vi "XY_plot_gnuplot.vi"(1 "Job Directory":path=path "/G4_2_HD/Users/paulhayden/Documents/Projects/Westlakes_resolution") -> (2 "Saved Automatically?":bool, 3 "Tex Info String":string="set term epslatex\nset output \"Plot.eps\"\nset xlabel '$Distance~(m)$'\nset ylabel '$DF~(s/m^3)\\times10^6$'\nset samples 1000\nset pointsize 1.00\nset title '$B38~Centreline~Glc$' 0, 0\nset size 0.75,0.9\n\n#set key 450, -2.5833\n unset key\nset label 1 '~~~~~~~~~~~Angle~(deg)~=~0' at -100, -2.58\nset label 2 '~~~~~~~~~~~Height~(m)~=~5' at -100, -3.27\n set xrange [0 : 500] \n# set autoscale x \n set yrange [0.10000 : 7]\n# set autoscale y \n\nplot \"B38_Centreline_Glc.dat\" index 0 using 1:2 axes x1y1 title '$File=B38R~DDD.xls$' with points 1 1, \\\n\"B38_Centreline_Glc.dat\" index 1 using 1:2 axes x1y1 title '$File=B38R~DDD~1.xls$' with points 1 3", 4 "Plot data file":path)   [LabVIEW 2022 SP3]
uses:
  Gnuplot_Label.ctl
  gnuplotScriptComponents/gridlines.ctl
  gnuplotScriptComponents/legendAppearance.ctl
  gnuplotScriptComponents/alignment.ctl
  gnuplotScriptComponents/legendProperties.ctl
  gnuplotScriptComponents/at.ctl
  <vilib>/Analysis/baseanly.llb/Mean (DBL).vi
  <vilib>/Utility/error.llb/Trim Whitespace One-Sided.vi
  Results_plotter_Global.vi
  Data plotting/subVIs/Plot_Values_Global.vi
  <vilib>/Analysis/NI_AALBase.lvlib
  <vilib>/Analysis/NI_AALPro.lvlib
panel:
  in  "Show Re-Run Gnuplot?":bool
  in  "Tab Control":T1(tab)
  in  "Plot Title":u16(ring) items=["Title String Only", "Date:Sortable:", "Run:Command:File", "Run:Start Time:", "Run:Description:", "Row:Number:", "Row:Type:", "Row:Start:(sec)", "Row:Comment:", "Timestamp::", "Config::", "Config:Num:", "Errata::", "Omit::", "WD::", "WD.Pt::", "WD.Pt.Cfg::", "Point:ID:", "Point:Row:", "Legend0::", "Downrange:Distance:(ft)", "Point:Height:Num", "Point:Column:", "Legend1::", "-:MeasuredVariables:-----------", "--:VelocityStats:--", "U_{dem}:Nominal:(m/s)", "U_{ref}::(m/s)", "\\overline{U}::(m/s)", "U:corr:(m/s)", "\\overline{V}::(m/s)", "\\overline{W}::(m/s)", "\\overline{|UV|}::(m/s)", "\\overline{|UW|}::(m/s)", "\\overline{|UVW|}::(m/s)", "\\overline{\\theta}::(deg)", "\\sigma^2(U)::(m/s)^2", "\\sigma^2(V)::(m/s)^2", "\\sigma^2(W)::(m/s)^2", "\\sigma^2(|UV|)::(m/s)^2", "\\sigma^2(|UW|)::(m/s)^2", "\\sigma^2(|UVW|)::(m/s)^2", "\\sigma^2(\\theta)::(deg^2)", "u'v'::(m^2/s^2)", "v'w'::(m^2/s^2)", "u'w'::(m^2/s^2)", "--:VelocityStatsEnd:--", "--:QAstats:--", "Omni:meanPSU:(V)", "Omni:varPSU:(V^2)", "Temp::(C)", "No Of:Measurement:Blocks", "No of:Analogue:Samples", "Flow:Measurement:Time", "Decimation::", "AFRaw:nGood:perDecBlock", "AFGoodV:nGood:perDecBlock", "AFGoodVP:nGood:perDecBlock", "AFRaw:nCone<58:deg", "AFRaw:nCone<90:deg", "AFRaw:Cone<58:deg", "AFRaw:Cone<90:deg", "Run:Messages:", "--:QAstatsEnd:--", "-:MeasuredVariablesEnd:-----------", "Max:(ConeAngle):(deg)", "Valid:AFReduction:Fraction", "Valid:Velocity:Fraction", "Valid:5hpPressure:Fraction", "-:LocationsStart:-------------", "Scale::", "Row:X:0", "X::(mm)", "Y::(mm)", "Z:(mm):", "U_{ref}:Z:(mm)", "Metadata:Motor:X", "Metadata:Motor:Y", "Metadata:Motor:Z", "-:LocationsEnd:-------------", "-:BLsetupBlock:------------", "BLS:Trip[1]:Ach(mm)", "BLS:Trip[2]:Ach(mm)", "BLS:Spires[1]:Ach(mm)", "BLS:Spires[2]:Ach(mm)", "BLS:Main[1]:Ach(mm)", "BLS:Main[2]:Ach(mm)", "BLS:Main[3]:Ach(mm)", "BLS:Boost[1]:Ach(mm)", "BLS:Boost[2]:Ach(mm)", "BLS:Boost[3]:Ach(mm)", "Main:Avg:(mm)", "Boost:Avg:(mm)", "FORMATTED:OUTPUT:BELOW-THIS-------------", "Configuration::", "Wind:Direction:(deg)", "BL:Setup:", "PointID::", "GDE:Uref:(m/s)", "Uref::(m/s)", "Mean:U:/U_{ref}", "Mean:V:/U_{ref}", "Mean:W:/U_{ref}", "Mean:|UV|:/U_{ref}", "Mean:|UW|:/U_ref", "Mean:|UVW|:/U_ref", "Yaw:(UV):(deg)", "TI:(U):(/U)", "TI:(U):(/|UV|)", "TI:(V):(/|UV|)", "TI:(W):(/|UW|)", "TI:(|UV|):(/|UV|)", "TI:(|UW|):(/|UW|)", "TI:(|UVW|):(/|UVW|)", "Velocity:Validation:(percent)", "Raw:Data:Filename", "FORMATTED:OUTPUT:ABOVE-THIS---------------", "Current:File:", "Current:Filepath:", "Template:File:Used", "Seconds:since:1st Jan", "Ramp:Request:0", "Ramp:Request:1", "Ramp:Request:2", "Ramp:Request:3", "Ramp:Request:4", "Ramp:Request:5", "Ramp:Request:6", "Ramp:Request:7", "Ramp:Request:8", "Ramp:Request:9", "Ramp:Request:10", "Ramp:Request:11", "Ramp:Request:12", "Point:Row:Column", "Number:of:Measurements"]
  in  "Plot Title":string
  in  "Added labels":i32[](listbox)
  in  "Show Labels?":bool
  in  "Summarise":u16(ring) items=["All Series", "\\overline{U} (m/s)", "GDE Uref (m/s)"]
  in  "X Log?":bool
  in  "Y Log?":bool
  in  "Ymin Val":dbl
  in  "Ymin":bool=TRUE
  in  "Xmin Val":dbl
  in  "Xmin":bool=TRUE
  in  "Xmax Val":dbl
  in  "Xmax":bool=TRUE
  in  "Ymax Val":dbl
  in  "Ymax":bool=TRUE
  in  "Major Gridlines":T2
  in  "Minor Gridlines":T2
  out "Time format?":bool
  in  "precision":string
  out "Profile offset":dbl
  in  "Offset?":bool
  in  "Mode":T3
  in  "Separation":dbl=1.2
  in  "Fit Line Width":i32=2
  in  "Fit type":T4(ring)
  in  "Put Coeff\nin Results file":bool
  in  "Analysis":T5(ring)
  in  "Wavelength?":bool
  in  "Auto Zp":bool=TRUE
  in  "Fixed Zp":dbl format="%.2f"
  in  "Something about fit..!":bool
  in  "Fit Line Type":i32=2
  in  "Current Fit Formula":string
  in  "Black and white?":bool
  in  "plot error bars?":bool
  in  "Plot style":u16[](array[ring])=[0, 0, 0, 0, 0, 0, 0, 0, 0, 0, 0] items=["points", "lines", "linespoints"]
  in  "Point Size":dbl=1.2 format="%.2f"
  in  "Graph Height":string="0.9"
  in  "Graph width":string="0.75"
  in  "Reverse order":bool
  in  "Appearance":T6
  in  "Show legend?":bool
  in  "Legend Position":u16(ring) items=["LabVIEW calculated", "top left", "top right", "bottom left", "bottom right", "below", "inside"]
  in  "Alignment":T7={"Horizontal"="center", "Vertical"="bottom"}
  in  "Save data analysis file":bool
  out "Path":path
  in  "Filename Max length":i32=28
  out "With legend":i32=580
  out "No Legend":i32=397
  out "No of Series":i32=2
  out "X location":dbl=-100.0
  out "Y location":dbl=-2.583333333333333
  out "Delta y":dbl=0.6900000000000001
  out "Extra range":dbl
  out "Final Title":string="B38 Centreline Glc"
  out "XY Graph":cluster{dbl[], dbl[]}[](graph)=[{[215.0, 270.0, 320.0, 445.0, 500.0, 500.0, 525.0, 600.0, 675.0, 750.0, 825.0, 900.0, 953.54, 960.0, 1010.0, 1060.0], [0.1374656, 0.6662545, 1.465458, 3.619824, 4.614524, 4.54365, 4.848976, 5.887329, 5.940571, 6.152151, 5.717487, 5.600293, 5.818368, 5.40069, 5.154843, 5.121789]}, {[100.0, 150.0, 215.0, 270.0, 320.0, 445.0, 525.0, 600.0, 675.0, 750.0, 825.0, 900.0, 960.0, 1010.0, 1060.0], [0.002314715, -0.00693192, 0.120417, 0.6880509, 1.519176, 3.513709, 5.065183, 6.116033, 6.096773, 5.938465, 5.593788, 5.5597, 5.387002, 5.304077, 4.887903]}]
  # "Scales"
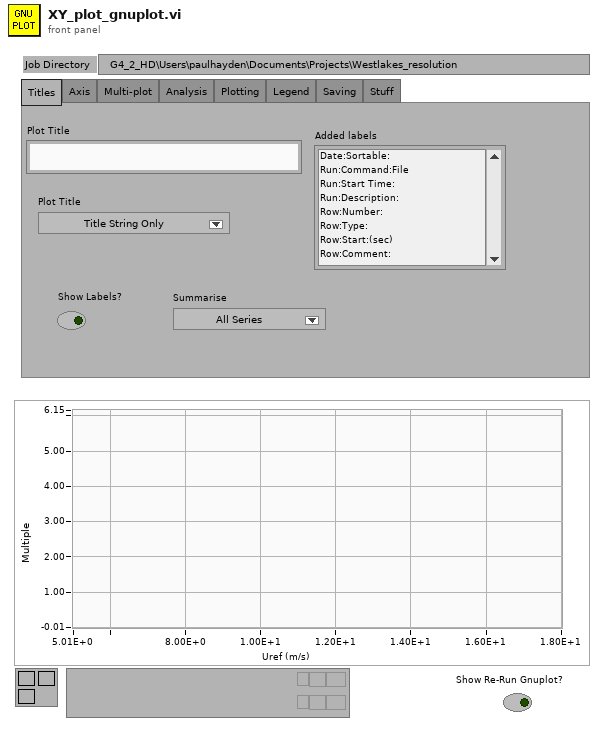
[diagram p1: front panel]
types:
  T1 = enum32{"Titles", "Axis", "Multi-plot", "Analysis", "Plotting", "Legend", "Saving", "Stuff"}
  T2 = typedef "gridlines.ctl" = enum16{"None", "X only", "Y only", "Both X and Y"}
  T3 = typedef "Gnuplot_Label.ctl" = enum16{"3 Labels per plot", "Only Center label", "Only Bottom Label"}
  T4 = enum16{"None", "Spline", "Linear", "2nd Poly", "3rd Poly", "4th Poly", "Gauss Lat", "Gauss vert", "Gauss Vert with 2 sig", "Guass glc"}
  T5 = enum16{"None", "% change", "Spectrum", "Norm Spec"}
  T6 = typedef "legendAppearance.ctl" = cluster{"layout":string, "text-sample order":string, "key order":string, "surroundingBox":string, "MaxRows":u32, "MaxCols":u32, "WidthAdjust":dbl}
  T7 = typedef "alignment.ctl" = cluster{"Horizontal":string, "Vertical":string}
  T8 = typedef "Error_bars.ctl" = cluster{"Upper":string[], "Lower":string[], "St Error":string[]}
  T9 = cluster{"Output":dbl[], "PercentageDifferenceArray":dbl[]}[]
  T10 = cluster{dbl[], "PercentageDifferenceArray":dbl[]}
  T11 = cluster{"Output":dbl[], "PercentageDifferenceArray":dbl[]}
  T12 = typedef "legendProperties.ctl" = cluster{"Appearance":T6, "Alignment":T7, "Location":string, "\"At\" location":T13}
  T13 = typedef "at.ctl" = cluster{"XcoordSys":string, "YcoordSys":string, "Xvalue":dbl, "Yvalue":dbl}
  T14 = typedef "RFP_Plot_Metadata.ctl" = cluster{"Row Number":i32[], "Error Bars":T15, "X Label":string, "Y Label":string, "Blanks NaNs":i32[]}
  T15 = typedef "Error_bars_index.ctl" = cluster{"Upper":i32, "Lower":i32, "St Error":i32}
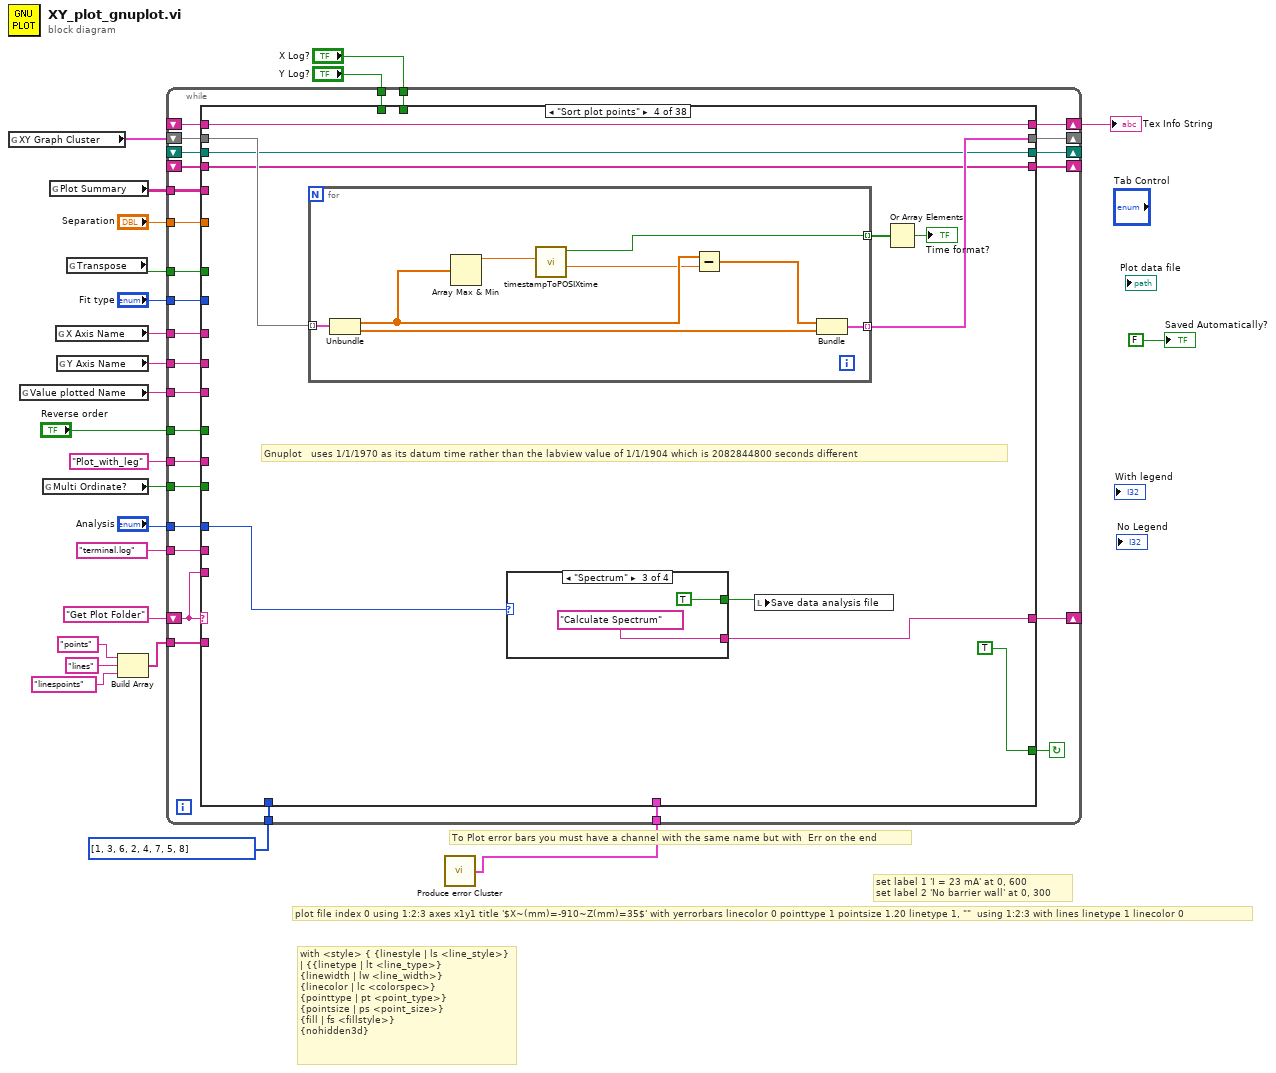
[diagram p0: block diagram]
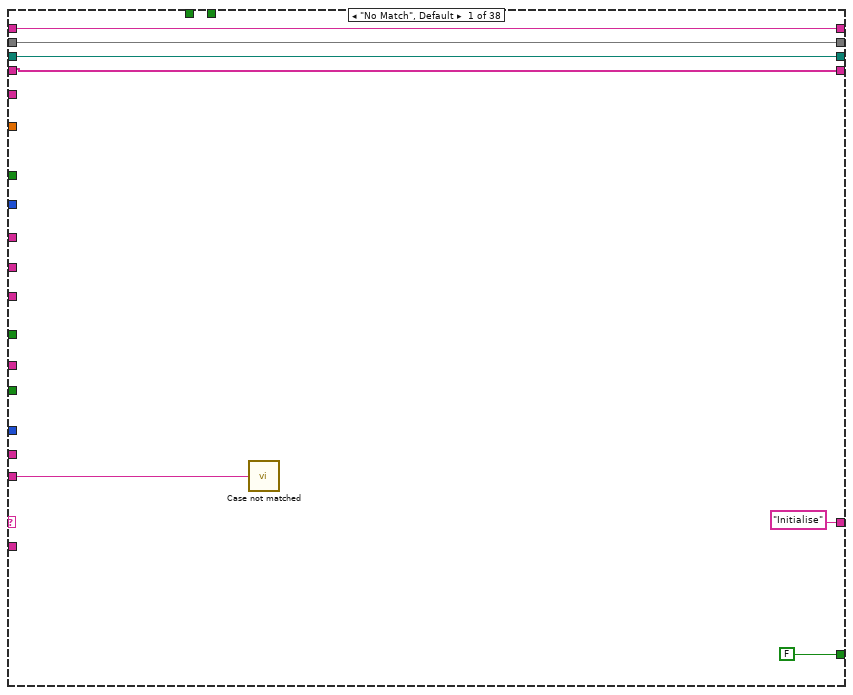
[diagram p2: hidden frame]
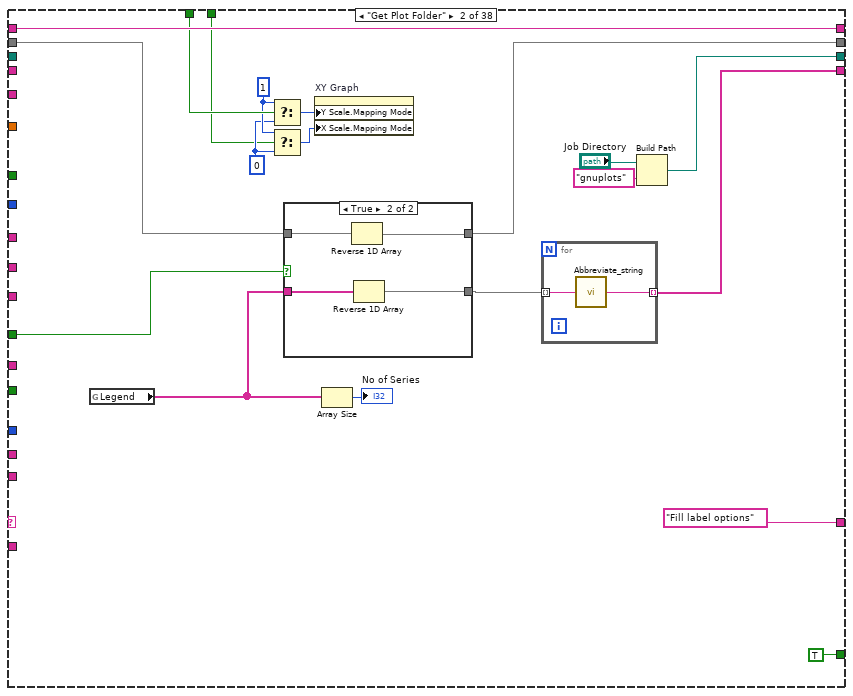
[diagram p3: hidden frame]
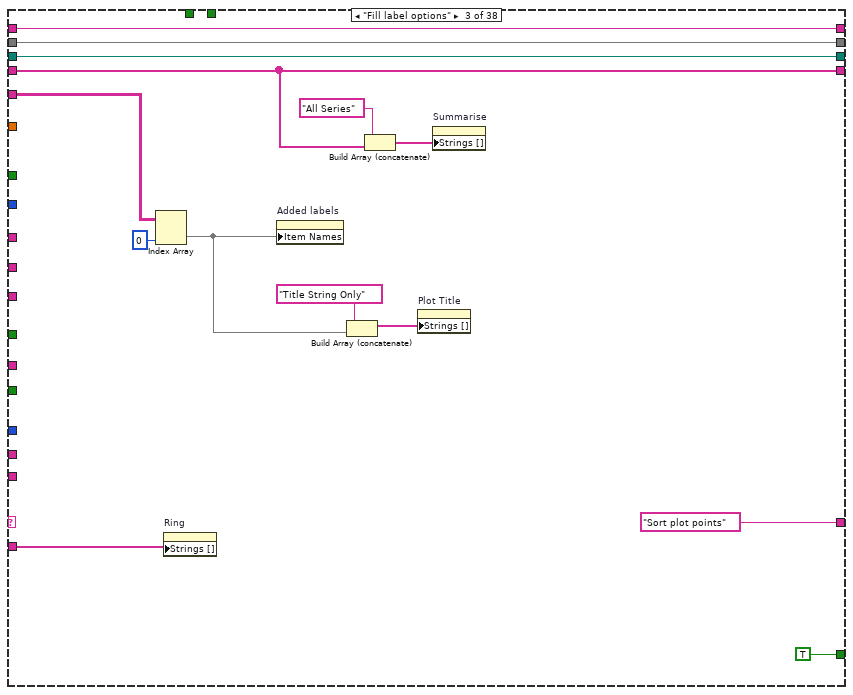
[diagram p5: hidden frame]
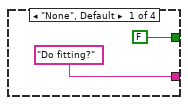
[diagram p6: hidden frame]
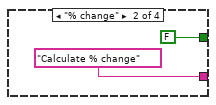
[diagram p7: hidden frame]
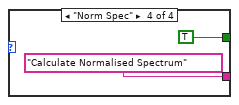
[diagram p8: hidden frame]
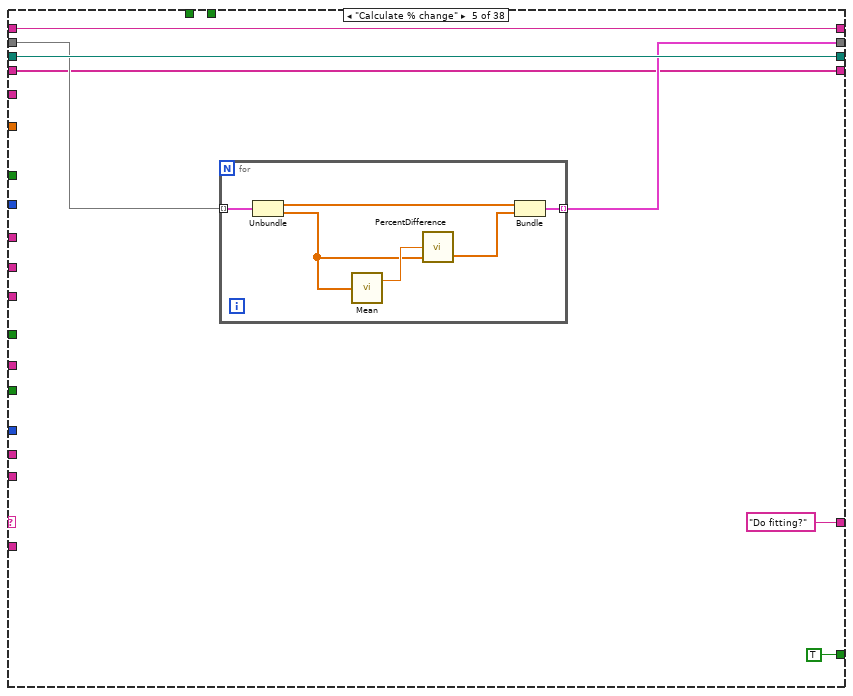
[diagram p9: hidden frame]
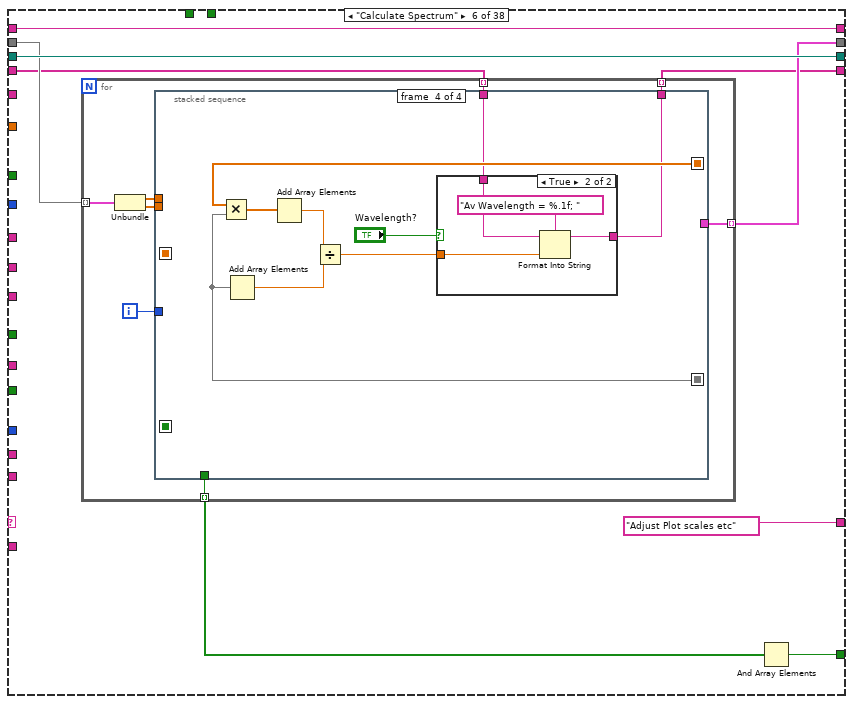
[diagram p10: hidden frame]
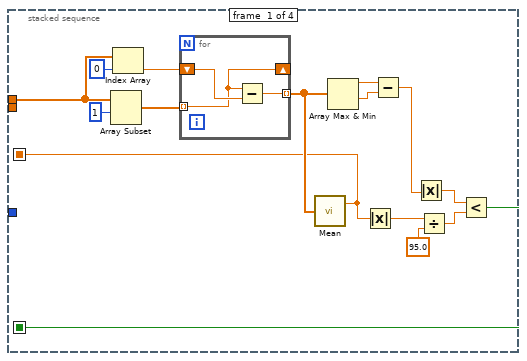
[diagram p11: hidden frame]
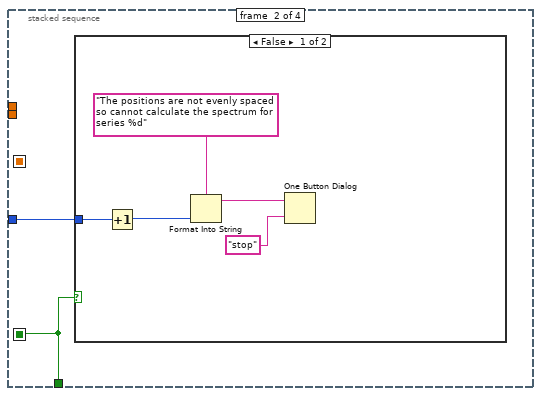
[diagram p12: hidden frame]
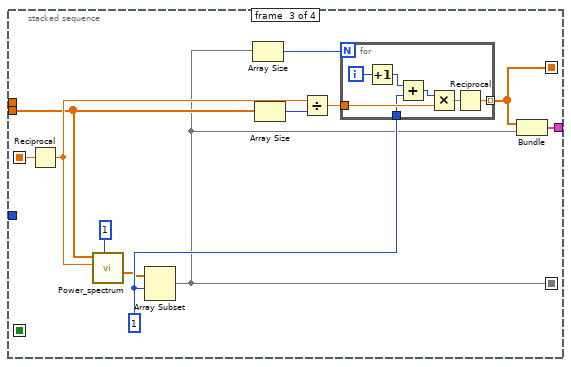
[diagram p14: hidden frame]
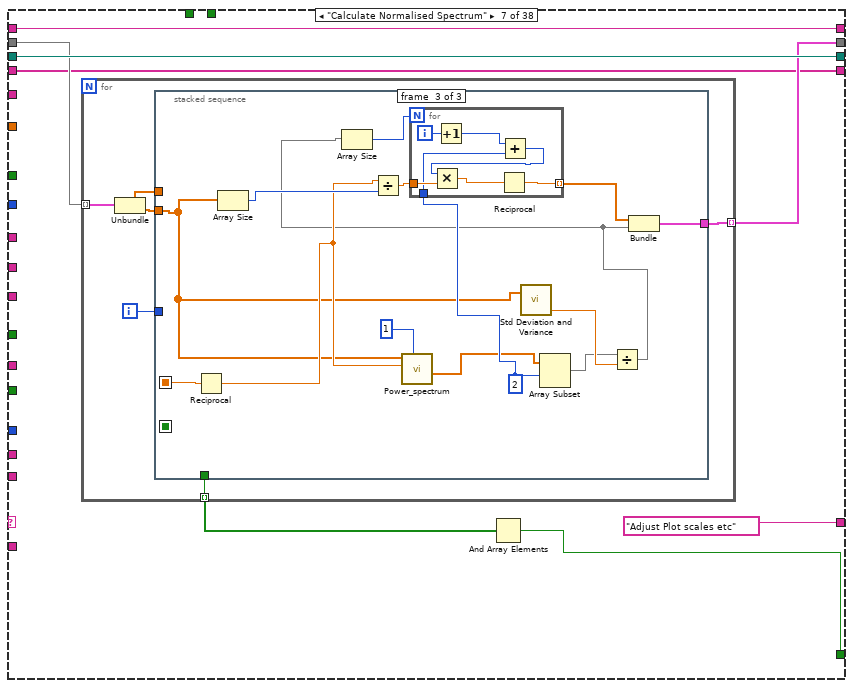
[diagram p16: hidden frame]
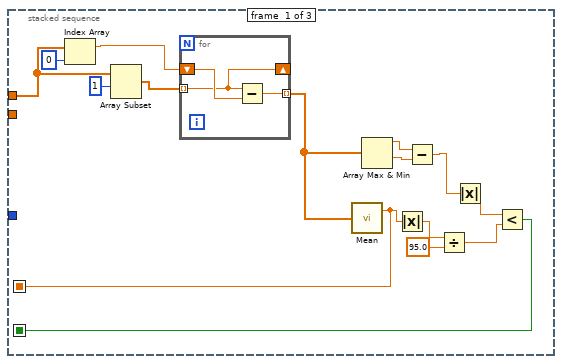
[diagram p17: hidden frame]
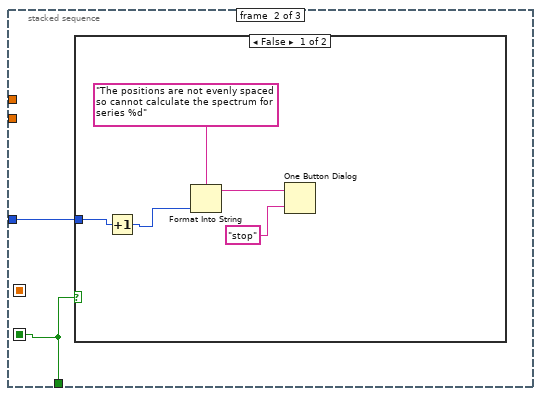
[diagram p18: hidden frame]
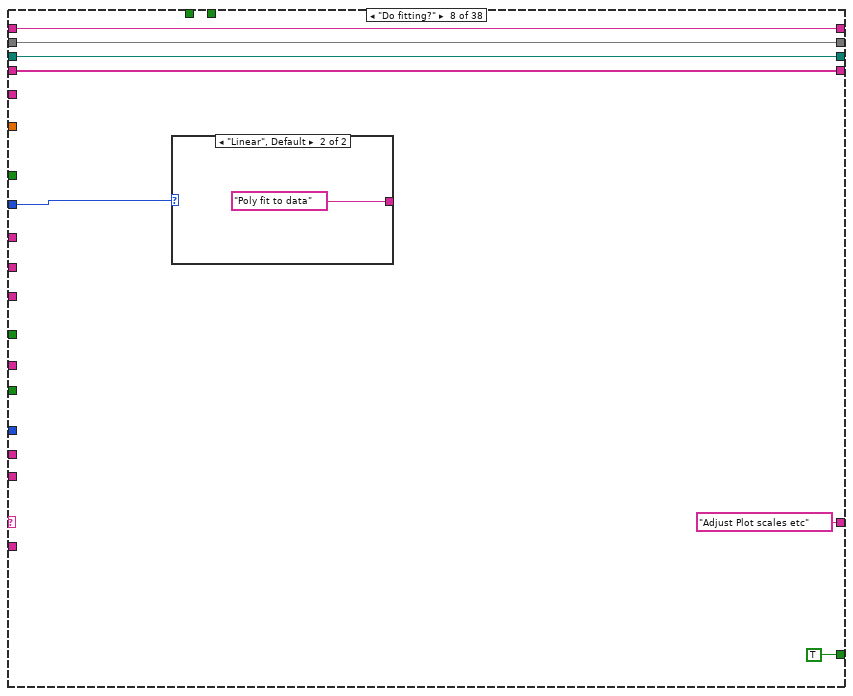
[diagram p20: hidden frame]
diagram:
  # "plot file index 0 using 1:2:3 axes x1y1 title '$X~(mm)=-910~Z(mm)=35$' with yerrorbars linecolor 0 pointtype 1 pointsize 1.20 linetype 1, \"\"  using 1:2:3 with lines linetype 1 linecolor 0"
  # "with <style> { {linestyle | ls <line_style>} \n| {{linetype | lt <line_type>} \n{linewidth | lw <line_width>} \n{linecolor | lc <colorspec>} \n{pointtype | pt <point_type>} \n{pointsize | ps <point_size>} \n{fill | fs <fillstyle>} \n{nohidden3d}"
  # "To Plot error bars you must have a channel with the same name but with  Err on the end"
  # "set label 1 'I = 23 mA' at 0, 600\nset label 2 'No barrier wall' at 0, 300"
  n1 = global read "Plot_Values_Global.vi" "XY Graph Cluster"() -> (w2:cluster{dbl[], dbl[]}[])
  n2 = global read "Results_plotter_Global.vi" "Value plotted Name"() -> (w20:string)
  n3 = global read "Results_plotter_Global.vi" "Multi Ordinate?"() -> (w4:bool)
  n4 = global read "Results_plotter_Global.vi" "Plot Summary"() -> (w23:string[][])
  n5 = global read "Results_plotter_Global.vi" "X Axis Name"() -> (w22:string)
  n6 = global read "Results_plotter_Global.vi" "Y Axis Name"() -> (w21:string)
  n7 = global read "Results_plotter_Global.vi" "Transpose"() -> (w5:bool)
  n8 = Build Array("points", "lines", "linespoints") -> (w10:string[])
  n9 = call "Produce error Cluster.vi"() -> ("Error Bar Cluster"=w3:T8[])  [unwired: 1 in]
  n10 = while {
    shift-left: "Get Plot Folder" -> [w50]
    shift-right: [w51] -> _
    tunnel: w23 -> [w49]
    shift-right: [w48] -> _
    shift-left: _ -> [w47]
    tunnel: "Analysis" -> [w46]
    tunnel: w22 -> [w45]
    tunnel: w21 -> [w44]
    tunnel: w20 -> [w43]
    shift-right: [w41] -> _
    shift-left: w2 -> [w42]
    shift-right: [w39] -> w18
    shift-left: _ -> [w40]
    tunnel: "Plot_with_leg" ("name or relative path") -> [w38]
    tunnel: "Fit type" -> [w37]
    shift-right: [w36] -> _
    shift-left: _ -> [w35]
    tunnel: "terminal.log" -> [w34]
    tunnel: w10 -> [w33]
    tunnel: i32[] [1, 3, 6, 2, 4, 7, 5, 8] ("Plot style") -> [w32]
    tunnel: "Separation" -> [w31]
    tunnel: "Y Log?" -> [w30]
    tunnel: w3 -> [w29]
    tunnel: "X Log?" -> [w28]
    tunnel: w5 -> [w27]
    tunnel: w4 -> [w26]
    tunnel: "Reverse order" -> [w25]
    stop <- w52 continue-if-true
    n11 = case shown="\"Sort plot points\"" w50 {
      tunnel: [FALSE TRUE TRUE ("Top Level") TRUE TRUE w143 w216 TRUE TRUE TRUE ("Top Level") TRUE ("Top Level") TRUE ("Top Level") TRUE ("Top Level") TRUE ("Top Level") TRUE ("Top Level") TRUE ("Top Level") TRUE ("Top Level") TRUE ("Top Level") TRUE ("Top Level") TRUE ("Top Level") w665 w738 TRUE ("Top Level") TRUE ("Top Level") TRUE ("Top Level") TRUE ("Top Level") TRUE ("Top Level") TRUE ("Top Level") TRUE ("Top Level") TRUE ("Top Level") TRUE ("Top Level") TRUE ("Top Level") TRUE ("Top Level") TRUE ("Top Level") TRUE ("Top Level") w1573 FALSE ("Top Level") FALSE ("Top Level")] -> w52
      tunnel: ["Initialise" "Fill label options" "Sort plot points" w104 "Do fitting?" "Adjust Plot scales etc" "Adjust Plot scales etc" "Adjust Plot scales etc" "Add fitted line styles" "Adjust Plot scales etc" w372 "Fill Second legend" "Fill Second legend" "Fill Second legend" "Calculate plot max and min values" "Sort out plot title" w557 w627 "Create plot directory" w651 w664 w737 w881 "Edit Legend names" w1069 "Labels?" ("t") "Labels?" ("t") w1236 w1247 "Plot Command" "Write gnuplot file" ("t") "Execute shell script" ("t") "Has pdf been generated?" ("t") w1549 "Input Fit Coefficients into results file?" "Read Fit Coefficients" ("t") "End" ("t") "End" ("t")] -> w51
      tunnel: w50 -> [w53 _ _ _ _ _ _ _ _ _ _ _ _ _ _ _ _ _ _ _ _ _ _ _ _ _ _ _ _ _ _ _ _ _ _ _ _ _]
      tunnel: w49 -> [_ _ w100 _ _ _ _ _ _ _ _ _ _ _ _ _ w566 _ _ _ w663 w736 _ _ _ _ _ _ w1246 _ _ _ _ _ _ _ _ _]
      tunnel: [w57 w75 w94 w108 w132 w148 w222 w281 w296 w357 w382 w408 w417 w429 w456 w490 w559 w628 w639 w653 w666 w739 w893 w935 w1084 w1155 w1213 w1243 w1253 w1379 w1411 w1534 w1542 w1555 w1566 w1577 w1599 w1731] -> w48
      tunnel: w47 -> [w57 _ w94 w108 w132 w148 w222 w281 w296 w357 w382 w408 w417 w429 w452 w490 w558 w624 w640 w648 w666 w739 w893 w935 w1084 w1155 w1213 w1243 w1253 w1379 w1411 w1534 w1542 w1555 w1566 w1577 w1599 w1731]
      tunnel: w46 -> [_ _ _ w105 _ _ _ _ _ _ w373 _ _ w423 _ _ _ w615 _ _ w659 w731 w890 _ _ _ _ _ _ _ _ _ _ _ _ _ _ _]
      tunnel: w45 -> [_ _ _ _ _ _ _ _ w287 _ _ w404 w416 _ _ _ _ _ _ _ w662 w735 w888 _ _ _ _ _ _ _ _ _ _ _ _ _ _ _]
      tunnel: w44 -> [_ _ _ _ _ _ _ _ w286 _ _ w403 w415 w428 _ _ _ _ _ _ w661 w734 w889 _ _ _ _ _ _ _ _ _ _ _ _ _ _ _]
      tunnel: w43 -> [_ _ _ _ _ _ _ _ _ _ _ _ _ _ _ _ _ _ _ _ w658 _ _ _ _ _ _ _ _ _ _ _ _ _ _ _ w1587 _]
      tunnel: w42 -> [w56 w71 w95 w110 w131 w147 w221 w277 w292 w356 w371 w407 w414 w427 w455 w487 w572 w626 w643 w656 w657 w733 w894 w923 w1079 w1150 w1209 w1240 w1248 w1380 w1412 w1540 w1547 w1562 w1571 w1581 w1592 w1736]
      tunnel: [w56 w70 w95 w109 w130 w146 w220 w277 w285 w356 w371 w407 w414 w427 w455 w487 w572 w626 w643 w656 w657 w730 w894 w923 w1079 w1150 w1209 w1240 w1248 w1380 w1412 w1540 w1547 w1562 w1571 w1581 w1592 w1736] -> w41
      tunnel: w40 -> [w55 w74 w96 w107 w129 w145 w219 w280 w295 w354 w374 w406 w413 w426 w454 w491 w567 w625 w642 w655 w667 w740 _ w933 w1083 w1121 w1189 w1231 w1250 w1377 w1409 w1529 w1545 w1560 w1569 w1579 w1602 w1734]
      tunnel: [w55 w74 w96 w107 w129 w145 w219 w280 w295 w354 w374 w406 w413 w426 w454 w491 w567 w625 w642 w655 w667 w740 w884 w931 w1083 w1118 w1188 w1230 w1251 w1373 w1408 w1529 w1545 w1560 w1569 w1579 w1602 w1734] -> w39
      tunnel: w38 -> [_ _ _ _ _ _ _ _ _ _ _ _ _ _ _ _ _ _ _ _ _ _ _ _ _ _ _ _ _ _ _ _ _ _ _ _ _ _]
      tunnel: w37 -> [_ _ _ _ _ _ _ w278 w294 _ w376 _ _ _ _ _ _ _ _ _ _ _ w882 w937 _ _ _ _ _ w1346 w1405 _ _ _ _ w1576 w1595 _]
      tunnel: [w54 w61 w92 w106 w128 w141 w218 w279 w289 w353 w378 w405 w412 w425 w453 w489 w571 w623 w641 w654 w660 w732 w892 w938 w1085 w1154 w1212 w1242 w1252 w1367 w1410 w1535 w1546 w1561 w1570 w1580 w1603 w1735] -> w36
      tunnel: w35 -> [w54 _ w92 w106 w128 w142 w218 w279 w290 w353 w378 w405 w412 w425 w453 w489 w571 w623 w641 w654 w660 w732 w892 w938 w1086 w1154 w1212 w1242 w1252 w1367 w1410 w1535 w1546 w1561 w1570 w1580 w1603 w1735]
      tunnel: w34 -> [_ _ _ _ _ _ _ _ _ _ _ _ _ _ _ _ _ _ _ _ _ _ _ _ _ _ _ _ _ _ _ _ w1541 _ _ _ _ w1729]
      tunnel: w33 -> [_ _ w90 _ _ _ _ _ _ _ _ _ _ _ _ _ _ _ _ _ _ _ _ _ _ _ _ _ _ _ _ _ _ _ _ _ _ _]
      tunnel: w32 -> [_ _ _ _ _ _ _ _ _ _ _ _ _ _ _ _ _ _ _ _ _ _ _ _ _ _ _ _ _ _ w1403 w1531 _ _ _ _ _ _]
      tunnel: w31 -> [_ _ _ _ _ _ _ _ _ _ _ _ _ _ _ _ _ _ _ _ _ w729 _ _ w1078 _ _ _ _ w1364 _ _ _ _ _ _ _ _]
      tunnel: w30 -> [_ w69 _ _ _ _ _ _ _ _ _ _ _ _ _ _ _ _ _ _ _ _ _ _ _ w1134 w1200 _ w1245 w1361 _ _ _ _ _ _ _ _]
      tunnel: w29 -> [_ _ _ _ _ _ _ _ _ _ _ _ _ _ _ w460 _ _ _ _ _ w728 _ _ _ _ _ _ _ _ w1402 _ _ _ _ _ _ _]
      tunnel: w28 -> [_ w64 _ _ _ _ _ _ _ _ _ _ _ _ _ _ _ _ _ _ _ _ _ _ _ w1131 _ _ w1244 w1356 _ _ _ _ _ _ _ _]
      tunnel: w27 -> [_ _ _ _ _ _ _ _ _ _ _ _ _ _ _ w458 _ _ _ _ _ w727 _ w924 _ _ _ _ _ w1351 w1399 _ _ _ _ _ _ _]
      tunnel: w26 -> [_ _ _ _ _ _ _ _ _ _ _ _ _ _ _ _ _ _ _ _ _ _ _ _ _ _ _ _ _ _ _ _ _ _ _ _ _ _]
      tunnel: w25 -> [_ w60 _ _ _ _ _ _ _ _ _ _ _ _ _ _ _ _ _ _ _ _ _ _ _ _ _ _ _ _ _ _ _ _ _ _ w1585 _]
      frame "No Match", Default {
        n12 = call "Case not matched.vi"("Case Name not Matched"=w53) -> ()
      }
      frame "Get Plot Folder" {
        w65 = u8 0 ("f")
        w66 = u8 1 ("Y Scale.Mapping Mode")
        n13 = global read "Results_plotter_Global.vi" "Legend"() -> (w63:string[])
        n14 = Select(t=w66, s=w69, f=w65) -> (s? t:f=w68:u8)
        n15 = Select(t=w66, s=w64, f=w65) -> (s? t:f=w67:u8)
        n16 = case shown="True" w60 {
          tunnel: w71 -> [w82 w86]
          tunnel: [w82 w85] -> w70
          tunnel: w63 -> [w81 w84]
          tunnel: [w81 w83] -> w62
          frame False {
          }
          frame True {
            n17 = Reverse 1D Array(array=w86) -> (reversed array=w85:T9)
            n18 = Reverse 1D Array(array=w84) -> (reversed array=w83:string[])
          }
        }
        n19 = property on="XY Graph" class="XYGraph (strict)"("Y Scale.Mapping Mode"=w68, "X Scale.Mapping Mode"=w67) -> ()  [unwired: 2 in, 2 out]
        n20 = Array Size(array=w63) -> (size(s)=→"No of Series":i32)
        n21 = for {
          tunnel: w62 -> [w80] mode=indexing
          tunnel: [w79] -> w61 mode=indexing
          n22 = call "Abbreviate_string.vi"("Input String"=w80) -> ("Output String"=w79:string)  [unwired: 2 in, 2 out]
        }
        n23 = Build Path(base path="Job Directory", name or relative path="gnuplots") -> (appended path=w75:path)
      }
      frame "Fill label options" {
        n24 = Index Array(array=w100, index (col)=0 ("disabled index (col)")) -> (element=w88:string[])  [unwired: 1 in]
        n25 = property on="Ring" class="Ring (strict)"("Strings []"=w90) -> ()  [unwired: 2 in, 2 out]
        n26 = property on="Added labels" class="LstBox (strict)"("Item Names"=w88) -> ()  [unwired: 2 in, 2 out]
        n27 = Build Array (concatenate)("Title String Only", w88) -> (w87:string[])
        n28 = Build Array (concatenate)("All Series", w92) -> (w93:string[])
        n29 = property on="Plot Title" class="Ring (strict)"("Strings []"=w87) -> ()  [unwired: 2 in, 2 out]
        n30 = property on="Summarise" class="Ring (strict)"("Strings []"=w93) -> ()  [unwired: 2 in, 2 out]
      }
      frame "Sort plot points" {
        # "Gnuplot   uses 1/1/1970 as its datum time rather than the labview value of 1/1/1904 which is 2082844800 seconds different"
        n31 = for {
          tunnel: w110 -> [w118] mode=indexing
          tunnel: [w119] -> w109 mode=indexing
          tunnel: [w112] -> w102 mode=indexing
          n32 = Unbundle(w118) -> ("Output"=w116:dbl[], "PercentageDifferenceArray"=w117:dbl[])
          n33 = Array Max & Min(array=w116) -> (max value=w114:dbl)  [unwired: 3 out]
          n34 = call "timestampToPOSIXtime.vi"("numberToTest"=w114) -> ("subtractForPOSIX"=w113:dbl, "looksLikeTimestamp"=w112:bool)  [unwired: 8 in, 1 out]
          n35 = Subtract(x=w116, y=w113) -> (x-y=w115:dbl[])
          n36 = Bundle(w115, "PercentageDifferenceArray"=w117) -> (w119:T10)  [unwired: 1 out]
        }
        n37 = case shown="\"Spectrum\"" w105 {
          tunnel: ["Do fitting?" "Calculate % change" "Calculate Spectrum" "Calculate Normalised Spectrum"] -> w104
          tunnel: [FALSE ("Save data analysis file") FALSE ("Save data analysis file") TRUE ("Save data analysis file") TRUE ("Save data analysis file")] -> w103
          frame "None", Default {
          }
          frame "% change" {
          }
          frame "Spectrum" {
          }
          frame "Norm Spec" {
          }
        }
        n38 = local write "Save data analysis file"(w103) -> ()
        n39 = Or Array Elements(Boolean array=w102) -> (logical OR=→"Time format?":bool)
      }
      frame "Calculate % change" {
        n40 = for {
          tunnel: w131 -> [w140] mode=indexing
          tunnel: [w138] -> w130 mode=indexing
          n41 = Unbundle(w140) -> ("Output"=w139:dbl[], "PercentageDifferenceArray"=w136:dbl[])
          n42 = call-poly <vilib>:"Mean.vi"("X"=w136) -> ("mean"=w137:dbl)  [unwired: 1 out]
          n43 = call "PercentDifference.vi"("CompareeArray"=w136, "Basis"=w137) -> ("PercentageDifferenceArray"=w135:dbl[])  [unwired: 1 in, 1 out]
          n44 = Bundle("Output"=w139, "PercentageDifferenceArray"=w135) -> (w138:T11)  [unwired: 1 out]
        }
      }
      frame "Calculate Spectrum" {
        n45 = for {
          tunnel: w147 -> [w156] mode=indexing
          tunnel: [w157] -> w146 mode=indexing
          tunnel: [w152] -> w144 mode=indexing
          tunnel: w142 -> [w151] mode=indexing
          tunnel: [w150] -> w141 mode=indexing
          i -> [w153]
          n46 = Unbundle(w156) -> ("Output"=w154:dbl[], "PercentageDifferenceArray"=w155:dbl[])
          n47 = stacked-sequence {
            seq-local: [w159 _ _ _] -> [_ _ w189 _]
            seq-local: [w158 _ _ _] -> [_ w176 _ _]
            seq-local: [_ _ w185 _] -> [_ _ _ w209]
            seq-local: [_ _ w184 _] -> [_ _ _ w210]
            tunnel: [_ _ w194 _] -> w157
            tunnel: w155 -> [_ _ w187 _]
            tunnel: w154 -> [w170 _ _ _]
            tunnel: w153 -> [_ w177 _ _]
            tunnel: [_ w176 _ _] -> w152
            tunnel: w151 -> [_ _ _ w205]
            tunnel: [_ _ _ w203] -> w150
            frame #0 {
              n48 = Array Subset(array=w170, index=1) -> (w168:dbl[])  [unwired: 1 in]
              n49 = Index Array(array=w170, index=0) -> (element=w169:dbl)
              n50 = for {
                shift-right: [w174] -> _
                shift-left: w169 -> [w175]
                tunnel: w168 -> [w174] mode=indexing
                tunnel: [w173] -> w165 mode=indexing
                n51 = Subtract(x=w174, y=w175) -> (x-y=w173:dbl)
              }
              n52 = call-poly <vilib>:"Mean.vi"("X"=w165) -> ("mean"=w159:dbl)  [unwired: 1 out]
              n53 = Array Max & Min(array=w165) -> (max value=w167:dbl, min value=w166:dbl)  [unwired: 2 out]
              n54 = Absolute Value(x=w159) -> (abs(x)=w162:dbl)
              n55 = Subtract(x=w167, y=w166) -> (x-y=w164:dbl)
              n56 = Absolute Value(x=w164) -> (abs(x)=w163:dbl)
              n57 = Divide(x=w162, y=95.0) -> (x/y=w160:dbl)
              n58 = Less?(x=w163, y=w160) -> (x < y?=w158:bool)
            }
            frame #1 {
              n59 = case shown="False" w176 {
                tunnel: w177 -> [w182 _]
                frame False {
                  n60 = Increment(x=w182) -> (x+1=w181:i32)
                  n61 = Format Into String(format string="The positions are not evenly spaced so cannot calculate the spectrum for series %d", w181) -> (resulting string=w179:string)  [unwired: 2 in, 1 out]
                  n62 = One Button Dialog(message=w179, button name ("OK")="stop") -> ()  [unwired: 1 out]
                }
                frame True {
                }
              }
            }
            frame #2 {
              w190 = 1 ("index")
              n63 = Reciprocal(x=w189) -> (1/x=w188:dbl)
              n64 = call "Power_spectrum.vi"("Block No"=1, "Sampling frequency"=w188, "U"=w187) -> ("SingleBlockSpectrum"=w183:dbl[])  [unwired: 2 in, 3 out]
              n65 = Array Subset(array=w183, index=w190) -> (w184:dbl[])  [unwired: 1 in]
              n66 = Array Size(array=w184) -> (size(s)=w193:i32)
              n67 = Array Size(array=w187) -> (size(s)=w191:i32)
              n68 = Divide(x=w188, y=w191) -> (x/y=w186:dbl)
              n69 = for {
                N: w193 -> [_]
                tunnel: [w198] -> w185 mode=indexing
                tunnel: w186 -> [w200]
                tunnel: w190 -> [w196]
                i -> [w201]
                n70 = Increment(x=w201) -> (x+1=w197:i32)
                n71 = Add(x=w197, y=w196) -> (x+y=w195:i32)
                n72 = Multiply(x=w195, y=w200) -> (x*y=w199:dbl)
                n73 = Reciprocal(x=w199) -> (1/x=w198:dbl)
              }
              n74 = Bundle(w185, w184) -> (w194:cluster{dbl[], dbl[]})  [unwired: 1 out]
            }
            frame #3 {
              n75 = Multiply(x=w209, y=w210) -> (x*y=w208:dbl[])
              n76 = Add Array Elements(numeric array=w210) -> (sum=w206:dbl)
              n77 = Add Array Elements(numeric array=w208) -> (sum=w207:dbl)
              n78 = Divide(x=w207, y=w206) -> (x/y=w204:dbl)
              n79 = case shown="True" "Wavelength?" {
                tunnel: w205 -> [w211 w215]
                tunnel: w204 -> [_ w214]
                tunnel: [w211 w212] -> w203
                frame False {
                }
                frame True {
                  n80 = Format Into String(format string="Av Wavelength = %.1f; ", initial string=w215, w214) -> (resulting string=w212:string)  [unwired: 1 in, 1 out]
                }
              }
            }
          }
        }
        n81 = And Array Elements(Boolean array=w144) -> (logical AND=w143:bool)
      }
      frame "Calculate Normalised Spectrum" {
        n82 = for {
          tunnel: w221 -> [w228] mode=indexing
          tunnel: [w229] -> w220 mode=indexing
          tunnel: [w224] -> w217 mode=indexing
          i -> [w225]
          n83 = Unbundle(w228) -> ("Output"=w226:dbl[], "PercentageDifferenceArray"=w227:dbl[])
          n84 = stacked-sequence {
            seq-local: [w231 _ _] -> [_ _ w262]
            seq-local: [w230 _ _] -> [_ w248 _]
            tunnel: [_ _ w268] -> w229
            tunnel: w227 -> [_ _ w260]
            tunnel: w226 -> [w242 _ _]
            tunnel: w225 -> [_ w249 _]
            tunnel: [_ w248 _] -> w224
            frame #0 {
              n85 = Index Array(array=w242, index=0) -> (element=w241:dbl)
              n86 = Array Subset(array=w242, index=1) -> (w240:dbl[])  [unwired: 1 in]
              n87 = for {
                shift-right: [w246] -> _
                shift-left: w241 -> [w247]
                tunnel: w240 -> [w246] mode=indexing
                tunnel: [w245] -> w237 mode=indexing
                n88 = Subtract(x=w246, y=w247) -> (x-y=w245:dbl)
              }
              n89 = call-poly <vilib>:"Mean.vi"("X"=w237) -> ("mean"=w231:dbl)  [unwired: 1 out]
              n90 = Array Max & Min(array=w237) -> (max value=w239:dbl, min value=w238:dbl)  [unwired: 2 out]
              n91 = Absolute Value(x=w231) -> (abs(x)=w234:dbl)
              n92 = Subtract(x=w239, y=w238) -> (x-y=w236:dbl)
              n93 = Divide(x=w234, y=95.0) -> (x/y=w232:dbl)
              n94 = Absolute Value(x=w236) -> (abs(x)=w235:dbl)
              n95 = Less?(x=w235, y=w232) -> (x < y?=w230:bool)
            }
            frame #1 {
              n96 = case shown="False" w248 {
                tunnel: w249 -> [w254 _]
                frame False {
                  n97 = Increment(x=w254) -> (x+1=w253:i32)
                  n98 = Format Into String(format string="The positions are not evenly spaced so cannot calculate the spectrum for series %d", w253) -> (resulting string=w251:string)  [unwired: 2 in, 1 out]
                  n99 = One Button Dialog(message=w251, button name ("OK")="stop") -> ()  [unwired: 1 out]
                }
                frame True {
                }
              }
            }
            frame #2 {
              w263 = 2 ("index")
              n100 = Reciprocal(x=w262) -> (1/x=w261:dbl)
              n101 = Array Size(array=w260) -> (size(s)=w264:i32)
              n102 = Divide(x=w261, y=w264) -> (x/y=w258:dbl)
              n103 = call "Power_spectrum.vi"("Block No"=1, "Sampling frequency"=w261, "U"=w260) -> ("SingleBlockSpectrum"=w255:dbl[])  [unwired: 2 in, 3 out]
              n104 = call <vilib>:"Std Deviation and Variance.vi"("X"=w260) -> ("variance"=w259:dbl)  [unwired: 1 in, 2 out]
              n105 = Array Subset(array=w255, index=w263) -> (w257:dbl[])  [unwired: 1 in]
              n106 = Divide(x=w257, y=w259) -> (x/y=w256:dbl[])
              n107 = Array Size(array=w256) -> (size(s)=w267:i32)
              n108 = for {
                N: w267 -> [_]
                tunnel: [w272] -> w266 mode=indexing
                tunnel: w258 -> [w274]
                tunnel: w263 -> [w270]
                i -> [w275]
                n109 = Increment(x=w275) -> (x+1=w271:i32)
                n110 = Add(x=w271, y=w270) -> (x+y=w269:i32)
                n111 = Multiply(x=w269, y=w274) -> (x*y=w273:dbl)
                n112 = Reciprocal(x=w273) -> (1/x=w272:dbl)
              }
              n113 = Bundle(w266, w256) -> (w268:cluster{dbl[], dbl[]})  [unwired: 1 out]
            }
          }
        }
        n114 = And Array Elements(Boolean array=w217) -> (logical AND=w216:bool)
      }
      frame "Do fitting?" {
        n115 = case shown="\"Linear\", Default" w278 {
          tunnel: ["Adjust Plot scales etc" "Poly fit to data"] -> _
          frame "None" {
          }
          frame "Linear", Default {
          }
        }
      }
      frame "Poly fit to data" {
        n116 = case shown="\"Linear\"" w294 {
          tunnel: [0 ("polynomial order") 1 ("polynomial order") 2 ("polynomial order") 3 ("polynomial order") 4 ("polynomial order")] -> w293
          frame "None", Default {
          }
          frame "Linear" {
          }
          frame "2nd Poly" {
          }
          frame "3rd Poly" {
          }
          frame "4th Poly" {
          }
        }
        n117 = for {
          tunnel: w292 -> [w316] mode=indexing
          tunnel: [w317] -> w291 mode=indexing
          tunnel: w293 -> [w315]
          tunnel: [w310] -> w288 mode=indexing
          tunnel: w287 -> [w309]
          tunnel: w286 -> [w308]
          w314 = 8  # Enhancement factor
          n118 = Unbundle(w316) -> ("Output"=w307:dbl[], "PercentageDifferenceArray"=w306:dbl[])
          n119 = call <vilib>:"General Polynomial Fit.vi"("Y"=w306, "polynomial order"=w315, "X"=w307) -> ("Polynomial Coefficients"=w304:dbl[])  [unwired: 9 in, 3 out]
          n120 = case shown="True" "Something about fit..!" {
            tunnel: [w320 w335] -> w311
            tunnel: [w331 w336] -> w310
            tunnel: w309 -> [w333 _]
            tunnel: w308 -> [w332 _]
            tunnel: w307 -> [w328 _]
            tunnel: w306 -> [w325 _]
            tunnel: w304 -> [_ w335]
            frame False {
              w327 = 0.99 ("Voltage")
              n121 = Build Array (concatenate)(nan ("Voltage"), w325) -> (w329:dbl[])
              n122 = Build Array (concatenate)(w327, w328) -> (w330:dbl[])
              n123 = call "Curve_Fit_ph.vi"("Values In"=w329, "No of points to fit (3)"=4, "Positions"=w330) -> ("Values Out"=w324:dbl[], "Polynomial Fit Coefficients"=w320:dbl[])  [unwired: 1 in]
              n124 = Index Array(array=w324, index=0) -> (element=w322:dbl)
              n125 = call "Number_2_string.vi"("precision"="2", "number"=w322) -> ("String"=w318:string)
              n126 = Format Into String(format string="When %s=%.2f ; %s=%s", w333, w327, w332, w318) -> (resulting string=w331:string)  [unwired: 2 in, 1 out]
            }
            frame True {
              n127 = for {
                shift-right: [w338] -> w336
                shift-left: "" -> [w339]
                tunnel: w335 -> [w342] mode=indexing
                i -> [w343]
                n128 = call "Number_2_string.vi"("number"=w342) -> ("String"=w340:string)  [unwired: 1 in]
                n129 = case shown="0, Default" w343 {
                  tunnel: [w344] -> w341
                  tunnel: w340 -> [w346]
                  frame 0, Default {
                    n130 = Concatenate Strings(w346, " ") -> (w344:string)
                  }
                }
                n131 = Concatenate Strings(w339, w341) -> (w338:string)
              }
            }
          }
          n132 = call "Enhance_No_of_points.vi"("Enhancement factor"=w314, "Input"=w307) -> ("Output"=w313:dbl[])  [unwired: 3 out]
          n133 = for {
            tunnel: w311 -> [w349]
            tunnel: w313 -> [w348] mode=indexing
            tunnel: [w347] -> w312 mode=indexing
            n134 = call "Polynomial_convert.vi"("Calib constants"=w349, "Voltage"=w348) -> ("Eng Values"=w347:dbl)  [unwired: 4 out]
          }
          n135 = Bundle("Output"=w313, w312) -> (w317:cluster{"Output":dbl[], dbl[]})  [unwired: 1 out]
        }
        n136 = Build Array (concatenate)(w290, w288) -> (w289:string[])
        n137 = Build Array (concatenate)(w292, w291) -> (w285:T9)
        n138 = local write "XY Graph"(w285) -> ()
      }
      frame "Add fitted line styles" {
        n139 = local read "No of Series"() -> (w350:i32)
        n140 = Array Subset(array=w353, index=w350) -> (w352:string[])  [unwired: 1 in]
        n141 = for {
          tunnel: w352 -> [w361] mode=indexing
          tunnel: u8 2 ("Plot.Plot Interpolation") -> [w367]
          tunnel: w350 -> [w363]
          i -> [w364]
          w369 = u32 0
          n142 = Concatenate Strings(w361, "  " ("string")) -> (w359:string)
          n143 = Add(x=w363, y=w364) -> (x+y=w362:i32)
          n144 = Quotient & Remainder(x=w364, y=4) -> (x-y*floor(x/y)=w365:i32)  [unwired: 1 out]
          n145 = property on="XY Graph" class="XYGraph (strict)"("Active Plot"=w362, "Plot.Plot Name"=w359, "Plot.Fill/Point Color"=w369, "Plot.Plot Color"=w369, "Plot.Point Style"=u8 0, "Plot.Line Style"=w365, "Plot.Plot Interpolation"=w367) -> ()  [unwired: 2 in, 2 out]
        }
      }
      frame "Adjust Plot scales etc" {
        w370 = u8[] [6, 1, 11, 2, 5, 13, 15, 10, 12, 14]  # pointStyles
        n146 = Greater Than 0?(x=w376) -> (x > 0?=w375:bool)
        n147 = Array Size(array=w378) -> (size(s)=w383:i32)
        n148 = local read "No of Series"() -> (w377:i32)
        n149 = property on="XY Graph" class="XYGraph (strict)"("Legend:Plots Shown"=w383) -> ()  [unwired: 2 in, 2 out]
        n150 = case shown="\"None\", Default" w373 {
          tunnel: ["Adjust plot scales2" "Show percentage change" ("t") "Set spectra axis" ("t") "Set spectra axis" ("t")] -> w372
          frame "None", Default {
          }
          frame "% change" {
          }
          frame "Spectrum" {
          }
          frame "Norm Spec" {
          }
        }
        n151 = Select(t=u8 2 ("Plot.Plot Interpolation"), s=w375, f=u8 0 ("Plot.Plot Interpolation")) -> (s? t:f=w379:u8)
        n152 = for {
          N: w377 -> [_]
          tunnel: w378 -> [w397] mode=indexing
          tunnel: w370 -> [w401]
          tunnel: w379 -> [w390]
          i -> [w400]
          w402 = u32 0
          n153 = String Length(string=w397) -> (length=w393:i32)
          n154 = Subtract(x=w393, y=2) -> (x-y=w391:i32)
          n155 = String Subset(string=w397, offset (0)=0, length (rest)=w391) -> (substring=w396:string)
          n156 = Concatenate Strings(w396, "  " ("string")) -> (w394:string)
          n157 = Index Array(array=w401, index=w400) -> (element=w399:u8)
          n158 = property on="XY Graph" class="XYGraph (strict)"("Active Plot"=w400, "Plot.Plot Name"=w394, "Plot.Fill/Point Color"=w402, "Plot.Plot Color"=w402, "Plot.Point Style"=w399, "Plot.Line Style"=u8 0, "Plot.Plot Interpolation"=w390) -> ()  [unwired: 2 in, 2 out]
        }
        "XY Graph" <- w371
      }
      frame "Adjust plot scales2" {
        n159 = property on="XY Graph" class="XYGraph (strict)"("X Scale.Name Label.Text"=w404, "Y Scale.Name Label.Text"=w403, "Cursor.Visible"=FALSE) -> ()  [unwired: 2 in, 2 out]
      }
      frame "Show percentage change" {
        n160 = Concatenate Strings(w415, " % Change" ("string")) -> (w418:string)
        n161 = property on="XY Graph" class="XYGraph (strict)"("X Scale.Name Label.Text"=w416, "Y Scale.Name Label.Text"=w418, "Cursor.Visible"=FALSE) -> ()  [unwired: 2 in, 2 out]
      }
      frame "Set spectra axis" {
        n162 = case shown="\"Spectrum\", Default" w423 {
          tunnel: [" Spectral Energy" ("string") " Normalised Spectral Energy" ("string")] -> w431
          frame "Spectrum", Default {
          }
          frame "Norm Spec" {
          }
        }
        n163 = Concatenate Strings(w428, w431) -> (w430:string)
        n164 = property on="XY Graph" class="XYGraph (strict)"("X Scale.Name Label.Text"="Wavelength [mm]", "Y Scale.Name Label.Text"=w430, "Cursor.Visible"=FALSE) -> ()  [unwired: 2 in, 2 out]
      }
      frame "Fill Second legend" {
        n165 = global read "Results_plotter_Global.vi" "Current Data Filenames"() -> (w441:string)
        n166 = call "Fast_string_Replace.vi"("Replace match with:"="_", "Input String"=w441, "matchThis"="[/]" ("regular expression")) -> ("Output String"=w445:string)  [unwired: 1 in, 1 out]
        n167 = call "Fast_string_Replace.vi"("Replace match with:"="_", "Input String"=w445, "matchThis"="__" ("regular expression")) -> ("Output String"=w442:string)  [unwired: 1 in, 1 out]
        n168 = call "Fast_string_Replace.vi"("Replace match with:"="", "Input String"=w442, "matchThis"=" " ("regular expression")) -> ("Output String"=w440:string)  [unwired: 1 in, 1 out]
        n169 = String Subset(string=w440, offset (0)=0, length (rest)=30 ("length (rest)")) -> (substring=w439:string)
        n170 = Build Path(base path=w452, name or relative path=w439) -> (appended path=w456:path)
      }
      frame "Calculate plot max and min values" {
        n171 = local read "plot error bars?"() -> (w459:bool)
        n172 = for {
          tunnel: w487 -> [w515] mode=indexing
          shift-right: [w512] -> w483
          shift-left: _ -> [w508]
          shift-right: [w511] -> w484
          shift-left: _ -> [w507]
          shift-right: [w510] -> w478
          shift-left: _ -> [w506]
          shift-right: [w509] -> w477
          shift-left: _ -> [w505]
          tunnel: w460 -> [w503]
          tunnel: w459 -> [w504]
          tunnel: w458 -> [w501]
          i -> [w502]
          n173 = Unbundle(w515) -> ("Output"=w514:dbl[], "PercentageDifferenceArray"=w513:dbl[])
          n174 = case shown="True" w504 {
            tunnel: w503 -> [_ w536]
            tunnel: w502 -> [_ w535]
            tunnel: [0.0 w531] -> w496
            frame False {
            }
            frame True {
              n175 = Index Array(array=w536, index=w535) -> (element=w534:T8)
              n176 = Unbundle(w534) -> ("Upper"=w533:string[])  [unwired: 2 out]
              n177 = Fract/Exp String To Number(string=w533) -> (number=w532:dbl[])  [unwired: 4 out]
              n178 = Array Max & Min(array=w532) -> (max value=w531:dbl)  [unwired: 3 out]
            }
          }
          n179 = Array Max & Min(array=w514) -> (max value=w494:dbl, min value=w492:dbl)  [unwired: 2 out]
          n180 = Array Max & Min(array=w513) -> (max value=w500:dbl, min value=w498:dbl)  [unwired: 2 out]
          n181 = case shown="True" w501 {
            tunnel: w500 -> [w522 w529]
            tunnel: [w521 w529] -> w499
            tunnel: w498 -> [w520 w528]
            tunnel: [w519 w528] -> w497
            tunnel: w496 -> [w518 w527]
            tunnel: [w517 w523] -> w495
            tunnel: w494 -> [w517 w526]
            tunnel: [w516 w524] -> w493
            tunnel: w492 -> [w516 w525]
            frame False {
              n182 = Subtract(x=w520, y=w518) -> (x-y=w519:dbl)
              n183 = Add(x=w522, y=w518) -> (x+y=w521:dbl)
            }
            frame True {
              n184 = Add(x=w526, y=w527) -> (x+y=w523:dbl)
              n185 = Subtract(x=w525, y=w527) -> (x-y=w524:dbl)
            }
          }
          n186 = case shown="1, Default" w502 {
            tunnel: [w540 w554] -> w512
            tunnel: w495 -> [w540 w553]
            tunnel: w493 -> [w539 w550]
            tunnel: [w539 w549] -> w511
            tunnel: [w538 w542] -> w510
            tunnel: w499 -> [w538 w545]
            tunnel: [w537 w541] -> w509
            tunnel: w497 -> [w537 w543]
            tunnel: w508 -> [_ w555]
            tunnel: w507 -> [_ w552]
            tunnel: w506 -> [_ w546]
            tunnel: w505 -> [_ w544]
            frame 0 {
            }
            frame 1, Default {
              n187 = Greater?(x=w546, y=w545) -> (0:w547:bool)
              n188 = Greater?(x=w555, y=w553) -> (0:w556:bool)
              n189 = Less?(x=w544, y=w543) -> (x < y?=w548:bool)
              n190 = Less?(x=w552, y=w550) -> (x < y?=w551:bool)
              n191 = Select(t=w546, s=w547, f=w545) -> (s? t:f=w542:dbl)
              n192 = Select(t=w544, s=w548, f=w543) -> (s? t:f=w541:dbl)
              n193 = Select(t=w555, s=w556, f=w553) -> (s? t:f=w554:dbl)
              n194 = Select(t=w552, s=w551, f=w550) -> (s? t:f=w549:dbl)
            }
          }
        }
        n195 = Subtract(x=w483, y=w484) -> (x-y=w485:dbl)
        n196 = Subtract(x=w478, y=w477) -> (x-y=w480:dbl)
        n197 = Multiply(x=w485, y=0.1) -> (x*y=w482:dbl)
        n198 = Multiply(x=w480, y=0.1) -> (x*y=w481:dbl)
        n199 = Add(x=w483, y=w482) -> (x+y=w470:dbl)
        n200 = Subtract(x=w484, y=w482) -> (x-y=w467:dbl)
        n201 = Add(x=w478, y=w481) -> (x+y=w463:dbl)
        n202 = Subtract(x=w477, y=w481) -> (x-y=w472:dbl)
        n203 = Select(t=w470, s="Xmax", f="Xmax Val") -> (s? t:f=w468:dbl)
        n204 = Select(t=w467, s="Xmin", f="Xmin Val") -> (s? t:f=w475:dbl)
        n205 = Select(t=w463, s="Ymax", f="Ymax Val") -> (s? t:f=w461:dbl)
        n206 = Select(t=w472, s="Ymin", f="Ymin Val") -> (s? t:f=w476:dbl)
        n207 = property on="XY Graph" class="XYGraph (strict)"("X Scale.Range:Maximum"=w468, "X Scale.Range:Minimum"=w475, "Y Scale.Range:Maximum"=w461, "Y Scale.Range:Minimum"=w476) -> ()  [unwired: 2 in, 2 out]
      }
      frame "Sort out plot title" {
        n208 = local read "Summarise"() -> (w570:u16)
        n209 = case shown="1, Default" "Plot Title" {
          selector: "Plot Title" -> [_ w588]
          tunnel: [w587 w594] -> w565
          tunnel: "Plot Title" -> [w587 w593]
          tunnel: w566 -> [_ w597]
          tunnel: w570 -> [_ w591]
          frame 0 {
          }
          frame 1, Default {
            n210 = Decrement(x=w588) -> (x-1=w596:u16)
            n211 = Add(x=w591, y=u16 2) -> (x+y=w590:u16)
            n212 = Index Array(array=w597, index (row)=w596, index (col)=w590) -> (element=w600:string)
            n213 = Empty String/Path?(string/path=w593) -> (empty?=w595:bool)
            n214 = call "Fast_string_Replace.vi"("Replace match with:"="~ ", "Input String"=w600, "matchThis"=":" ("regular expression")) -> ("Output String"=w599:string)  [unwired: 1 in, 1 out]
            n215 = call <vilib>:"Trim Whitespace.vi"("string"=w599) -> ("trimmed string"=w598:string)  [unwired: 1 in]
            n216 = call "Fast_string_Replace.vi"("Replace match with:"="~", "Input String"=w598, "matchThis"="_" ("regular expression")) -> ("Output String"=w589:string)  [unwired: 1 in, 1 out]
            n217 = case shown="False" w595 {
              tunnel: [w606 w609] -> w594
              tunnel: w589 -> [w608 w609]
              tunnel: w593 -> [w607 _]
              frame False {
                n218 = Concatenate Strings(w607, " " ("string"), w608) -> (w606:string)
              }
              frame True {
              }
            }
          }
        }
        n219 = case shown="False" "Show Labels?" {
          tunnel: w566 -> [w582 _]
          tunnel: w565 -> [w585 w586]
          tunnel: [w583 w586] -> w564
          frame False {
            n220 = local read "Added labels"() -> (w584:i32[])
            n221 = Concatenate Strings(w585, "         " ("string")) -> (w581:string)
            n222 = call "DistillTitle.vi"("Plot Summary in"=w582, "Show Channels with range of Values?"=FALSE, "Indices to include in Page Title"=w584, "String in"=w581) -> ("String out"=w583:string)  [unwired: 6 in, 1 out]
          }
          frame True {
          }
        }
        "Final Title" <- w564
        n223 = Current VI's Path() -> (path=w562:path)
        n224 = call "Running_as_top_level.vi"("Vi path name"=w562) -> ("Top Level"=w560:bool)  [unwired: 1 out]
        n225 = case shown="True" w560 {
          tunnel: [w574 w577] -> w559
          tunnel: w558 -> [w574 _]
          tunnel: ["Get Filename" ("t") "Create plot directory"] -> w557
          frame False {
          }
          frame True {
            n226 = local read "Path"() -> (w576:path)
            n227 = Strip Path(path=w576) -> (name=w575:string)  [unwired: 1 out]
            n228 = Build Path(base path=w576, name or relative path=w575) -> (appended path=w577:path)
          }
        }
      }
      frame "Get Filename" {
        n229 = local read "Final Title"() -> (w613:string)
        n230 = case shown="\"% change\"" w615 {
          tunnel: ["" "Per_" "Spec_" "N_Spec_"] -> w614
          frame "None" {
          }
          frame "% change" {
          }
          frame "Spectrum" {
          }
          frame "Norm Spec" {
          }
        }
        n231 = Concatenate Strings(w614, w613) -> (w610:string)
        n232 = String Length(string=w613) -> (length=w612:i32)
        n233 = case shown="0" w612 {
          tunnel: [w630 w631] -> w611
          tunnel: w610 -> [w630 w633]
          frame 0 {
          }
          frame 1, Default {
            n234 = Concatenate Strings(w633, "_") -> (w631:string)
          }
        }
        n235 = call "Auto_filename.vi"("Filename Max length"="Filename Max length", "Prefix"=w611) -> ("Filename"=w617:string)
        n236 = Build Path(base path=w624, name or relative path=w617) -> (appended path=w621:path)
        n237 = File/Directory Info(path=w621) -> (error out=w622:errorcluster)  [unwired: 1 in, 6 out]
        n238 = Build Path(base path=w621, name or relative path=w617) -> (appended path=w628:path)
        n239 = Unbundle By Name(w622) -> ("status"=w620:bool)
        n240 = Select(t="Create plot directory", s=w620, f="Find a unique name") -> (s? t:f=w627:string)
      }
      frame "Find a unique name" {
        n241 = call "FindUniqueName.vi"("Max Length"=27, "PathIn"=w640) -> ("UniquedPath"=w639:path)  [unwired: 9 in]
      }
      frame "Create plot directory" {
        n242 = Strip Path(path=w648) -> (stripped path=→"Path":path)  [unwired: 1 out]
        n243 = call "Create_directory_path.vi"("Path name"=w648) -> ("Path name Out"=w653:path)  [unwired: 2 in, 1 out]
        n244 = Select(t="Save data analysis file", s="Save data analysis file", f="Save .dat file") -> (s? t:f=w651:string)
      }
      frame "Save data analysis file" {
        n245 = stacked-sequence {
          seq-local: [w668 _ _] -> [_ _ w712]
          seq-local: [_ w684 _] -> [_ _ w710]
          tunnel: w666 -> [_ _ w723]
          tunnel: [_ _ TRUE ("Top Level")] -> w665
          tunnel: [_ _ "Save .dat file"] -> w664
          tunnel: w663 -> [w671 w686 _]
          tunnel: w662 -> [_ _ _]
          tunnel: w661 -> [_ _ _]
          tunnel: w657 -> [_ w687 _]
          tunnel: w659 -> [w675 _ _]
          tunnel: w658 -> [w674 _ _]
          frame #0 {
            n246 = case shown="\"Norm Spec\"" w675 {
              tunnel: w674 -> [w678 w682]
              tunnel: [w677 w681] -> w673
              tunnel: ["Wavelength::[mm]" "Wavelength::[mm]"] -> w672
              frame "Spectrum", Default {
                n247 = Concatenate Strings(w678, ":Spectral:Energy") -> (w677:string)
              }
              frame "Norm Spec" {
                n248 = Concatenate Strings(w682, ":Normalised Spectral:Energy") -> (w681:string)
              }
            }
            n249 = Index Array(array=w671, index (col)=0 ("disabled index (col)")) -> (element=w669:string[])  [unwired: 1 in]
            n250 = Build Array (concatenate)(w672, w673, w669) -> (w668:string[])
          }
          frame #1 {
            n251 = for {
              tunnel: w687 -> [w698] mode=indexing
              tunnel: w686 -> [w695]
              shift-right: [w689] -> w684
              shift-left: string[][] [] -> [w688]
              i -> [w693]
              n252 = Unbundle(w698) -> ("Output"=w697:dbl[], "PercentageDifferenceArray"=w696:dbl[])
              n253 = Add(x=3 ("disabled index (col)"), y=w693) -> (x+y=w692:i32)
              n254 = Index Array(array=w695, index (col)=w692) -> (element=w691:string[])  [unwired: 1 in]
              n255 = for {
                tunnel: w697 -> [w704] mode=indexing
                tunnel: w696 -> [w703] mode=indexing
                tunnel: w691 -> [w700]
                tunnel: [w699] -> w690 mode=indexing
                n256 = call "Number_2_string.vi"("number"=w704) -> ("String"=w702:string)  [unwired: 1 in]
                n257 = call "Number_2_string.vi"("number"=w703) -> ("String"=w701:string)  [unwired: 1 in]
                n258 = Build Array (concatenate)(w702, w701, w700) -> (w699:string[])
              }
              n259 = Build Array (concatenate)(w688, w690) -> (w689:string[][])
            }
          }
          frame #2 {
            w719 = FALSE  # Append last row only
            w718 = FALSE  # exists?
            n260 = Strip Path(path=w723) -> (stripped path=w724:path, name=w726:string)
            n261 = Array Size(array=w710) -> (size(s)=w709:i32[])
            n262 = Concatenate Strings(w726, ".xls" ("string")) -> (w725:string)
            n263 = Index Array(array=w709, index=0) -> (element=w707:i32)
            n264 = Build Path(base path=w724, name or relative path=w725) -> (appended path=w713:path)
            n265 = Initialize Array("", w707) -> (w706:string[])
            n266 = Build Array (concatenate)(w706, w710) -> (w711:string[][])
            n267 = Initialize Array("", 10 ("Dimension Size")) -> (w717:string[])
            n268 = call "Asterisk_header.vi"("Channel names"=w717) -> ("Header string"=w714:string)
            n269 = call "Write_Ch_data_file.vi"("Append last row only"=w719, "Header string"=w714, "exists?"=w718, "Channel Values"=w711, "Channel names"=w712, "Filename"=w713) -> ()  [unwired: 1 in, 5 out]
          }
        }
      }
      frame "Save .dat file" {
        n270 = stacked-sequence {
          seq-local: [w741 _ _ _ _] -> [_ _ _ _ w861]
          seq-local: [_ w767 _ _ _] -> [_ _ _ _ w862]
          seq-local: [_ _ _ w800 _] -> [_ _ _ _ w863]
          seq-local: [_ _ w784 _ _] -> [_ _ _ w798 _]
          seq-local: [_ _ w776 _ _] -> [_ _ _ w795 _]
          seq-local: [_ _ w778 _ _] -> [_ _ _ w794 _]
          tunnel: w739 -> [_ _ _ _ w866]
          tunnel: [_ _ _ _ TRUE ("Top Level")] -> w738
          tunnel: [_ _ _ _ "Gnuplot script Start"] -> w737
          tunnel: w736 -> [w746 _ _ _ _]
          tunnel: w735 -> [_ w770 _ _ _]
          tunnel: w734 -> [_ w766 _ _ _]
          tunnel: w733 -> [_ _ _ w802 _]
          tunnel: w732 -> [_ _ _ w799 _]
          tunnel: w731 -> [_ w764 _ _ _]
          tunnel: [_ _ _ w797 _] -> w730
          tunnel: w729 -> [_ _ w782 _ _]
          tunnel: w728 -> [_ _ _ w796 _]
          tunnel: w727 -> [_ _ w779 _ _]
          frame #0 {
            n271 = Array Subset(array=w746, length (col)=3 ("length")) -> (w744:string[][])  [unwired: 3 in]
            n272 = Build Array("Column Name", "Numeric Tolerance", "Range of Values") -> (w750:string[])
            n273 = Build Array (concatenate)(w750, w744) -> (w742:string[][])
            n274 = for {
              shift-right: [w754] -> w741
              shift-left: "" -> [w751]
              tunnel: w742 -> [w755] mode=indexing
              n275 = for {
                shift-right: [w756] -> w753
                shift-left: w751 -> [w763]
                tunnel: w755 -> [w757] mode=indexing
                i -> [w762]
                n276 = Equal To 0?(x=w762) -> (x = 0?=w761:bool)
                n277 = Select(t="#", s=w761, f="\t") -> (s? t:f=w758:string)
                n278 = Concatenate Strings(w763, w758, w757) -> (w756:string)
              }
              n279 = Concatenate Strings(w753, "\n") -> (w754:string)
            }
          }
          frame #1 {
            w768 = "\n"
            n280 = case shown="\"% change\"" w764 {
              tunnel: w766 -> [w772 w774]
              tunnel: [w772 w773] -> w765
              frame "None", Default {
              }
              frame "% change" {
                n281 = Concatenate Strings(w774, " %" ("string")) -> (w773:string)
              }
            }
            n282 = Concatenate Strings(w768, w768, "#" ("string"), w770, "\t", w765, w768, w768) -> (w767:string)
          }
          frame #2 {
            n283 = global read "Results_plotter_Global.vi" "Precision"() -> (w781:string[])
            n284 = global read "Results_plotter_Global.vi" "Absisca"() -> (w780:i32)
            n285 = case shown="True" "Offset?" {
              tunnel: [0.0 w792] -> w785
              frame False {
              }
              frame True {
                n286 = property on="XY Graph" class="XYGraph (strict)"() -> ("Y Scale.Range:Maximum"=w791:dbl, "Y Scale.Range:Minimum"=w793:dbl)  [unwired: 2 in, 2 out]
                n287 = Subtract(x=w791, y=w793) -> (x-y=w792:dbl)
              }
            }
            "Profile offset" <- w785
            n288 = Index Array(array=w781, index=w780) -> (element=w777:string)
            n289 = case shown="False" w779 {
              tunnel: ["" w789] -> w778
              tunnel: w777 -> [w786 w789]
              tunnel: [w786 ""] -> w776
              frame False {
              }
              frame True {
              }
            }
            n290 = Multiply(x=w785, y=w782) -> (x*y=w784:dbl)
          }
          frame #3 {
            n291 = for {
              tunnel: w802 -> [w829] mode=indexing
              shift-right: [w828] -> w800
              shift-left: "" -> [w819]
              tunnel: w799 -> [w817] mode=indexing
              tunnel: w798 -> [w814]
              tunnel: [w820] -> w797 mode=indexing
              tunnel: w796 -> [w807] mode=indexing
              tunnel: w795 -> [w804]
              tunnel: w794 -> [w803]
              i -> [w824]
              w827 = "\n"
              n292 = Multiply(x=w814, y=w824) -> (x*y=w809:dbl)
              n293 = Unbundle(w829) -> ("Output"=w822:dbl[], "PercentageDifferenceArray"=w823:dbl[])
              n294 = Negate(x=w809) -> (-x=w808:dbl)
              n295 = call "Number_2_string.vi"("number"=w808) -> ("String"=w816:string)  [unwired: 1 in]
              n296 = Format Into String(format string="\\t%s\\tPlot offset", w816) -> (resulting string=w812:string)  [unwired: 2 in, 1 out]
              n297 = Equal To 0?(x=w809) -> (x = 0?=w813:bool)
              n298 = Select(t="", s=w813, f=w812) -> (s? t:f=w810:string)
              n299 = Unbundle(w807) -> ("Upper"=w806:string[])  [unwired: 2 out]
              n300 = for {
                tunnel: w822 -> [w848] mode=indexing
                shift-right: [w837] -> w826
                shift-left: "" -> [w838]
                tunnel: w823 -> [w845] mode=indexing
                tunnel: w809 -> [w844]
                tunnel: [w843] -> w821 mode=indexing
                tunnel: w806 -> [w840]
                shift-right: [w836] -> _
                shift-left: string[] [] -> [w835]
                tunnel: w804 -> [w832]
                tunnel: w803 -> [w831]
                i -> [w841]
                w842 = "\t"
                n301 = Subtract(x=w845, y=w844) -> (x-y=w843:dbl)
                n302 = call "Number_2_string.vi"("precision"=w832, "number"=w848) -> ("String"=w847:string)
                n303 = call "Number_2_string.vi"("precision"=w831, "number"=w843) -> ("String"=w846:string)
                n304 = Index Array(array=w840, index=w841) -> (element=w839:string)
                n305 = Concatenate Strings(w847, w842, w846, w842, w839, "\n") -> (w834:string)
                n306 = Search 1D Array(1D array=w835, element=w834) -> (index of element=w833:i32)  [unwired: 1 in]
                n307 = case shown="-1" w833 {
                  tunnel: w838 -> [w850 w855]
                  tunnel: [w850 w854] -> w837
                  tunnel: w834 -> [_ w851]
                  tunnel: w835 -> [w849 w853]
                  tunnel: [w849 w852] -> w836
                  frame 0, Default {
                  }
                  frame -1 {
                    n308 = Concatenate Strings(w855, w851) -> (w854:string)
                    n309 = Build Array (concatenate)(w853, w851) -> (w852:string[])
                  }
                }
              }
              n310 = Bundle("Output"=w822, w821) -> (w820:cluster{"Output":dbl[], dbl[]})  [unwired: 1 out]
              n311 = Concatenate Strings(w819, "#", w817, w810, w827, w826, w827, w827) -> (w828:string)
            }
          }
          frame #4 {
            w858 = FALSE  # advisory dialog? (display:T)
            w859 = FALSE  # append to file? (new file:F)
            n312 = Strip Path(path=w866) -> (stripped path=w867:path, name=w869:string)
            n313 = Concatenate Strings(w861, w862, w863) -> (w860:string)
            n314 = Concatenate Strings(w869, ".dat" ("string")) -> (w868:string)
            n315 = Build Path(base path=w867, name or relative path=w868) -> (appended path=w857:path)
            n316 = call "Write_Characters_To_File.vi"("file path (dialog if empty)"=w857, "advisory dialog? (display:T)"=w858, "character string"=w860, "append to file? (new file:F)"=w859) -> ()  [unwired: 1 in, 4 out]
          }
        }
      }
      frame "Gnuplot script Start" {
        n317 = case shown="\"None\", Default" w890 {
          tunnel: w889 -> [w907 w910 w914 w918]
          tunnel: [w907 w909 w913 w917] -> w877
          tunnel: [w906 w908 "Wavelength [mm]" ("X Axis Name") "Wavelength [mm]" ("X Axis Name")] -> w876
          tunnel: w888 -> [w906 w908 _ _]
          frame "None", Default {
          }
          frame "% change" {
            n318 = Concatenate Strings(w910, " % change" ("string")) -> (w909:string)
          }
          frame "Spectrum" {
            n319 = Concatenate Strings(w914, " Spectral energy" ("string")) -> (w913:string)
          }
          frame "Norm Spec" {
            n320 = Concatenate Strings(w918, " Normalised Spectral Energy" ("string")) -> (w917:string)
          }
        }
        n321 = local read "Final Title"() -> (w878:string)
        n322 = case shown="\"Linear\", Default" w882 {
          tunnel: [w897 w899 "Calculate fit parameters"] -> w881
          tunnel: "Edit Legend names" -> [w897 w899 _]
          tunnel: [w896 w898 "set parametric\nset samples 1000\n"] -> w870
          tunnel: "" -> [w896 w898 _]
          frame "None" {
          }
          frame "Spline" {
          }
          frame "Linear", Default {
          }
        }
        n323 = call "setTerm.vi"() -> ("String out"=w875:string)  [unwired: 10 in, 1 out]
        n324 = call "TypesetInsideMathmode.vi"("DirtyString"=w876) -> ("Mathmode String"=w872:string)  [unwired: 8 in, 2 out]
        n325 = call "TypesetInsideMathmode.vi"("DirtyString"=w877) -> ("Mathmode String"=w871:string)  [unwired: 8 in, 2 out]
        n326 = call "TypesetInsideMathmode.vi"("DirtyString"=w878) -> ("Mathmode String"=w874:string)  [unwired: 8 in, 2 out]
        n327 = local read "Time format?"() -> (w883:bool)
        n328 = call "setTitle.vi"("Title"=w874, "String in"=w875) -> ("String out"=w873:string)  [unwired: 8 in, 1 out]
        n329 = Format Into String(format string="set xlabel '%s'\nset ylabel '%s'\nset size %s,%s\n%s", initial string=w873, w872, w871, "Graph width", "Graph Height", w870) -> (resulting string=w885:string)  [unwired: 1 in, 1 out]
        n330 = case shown="True" w883 {
          tunnel: w885 -> [w902 w904]
          tunnel: [w902 w903] -> w884
          frame False {
          }
          frame True {
            n331 = Concatenate Strings(w904, "\nset xdata time\nset timefmt \"%s\"\nset format  x \"%H:%M\\n%Y-%m-%d\"\n") -> (w903:string)
          }
        }
      }
      frame "Calculate fit parameters" {
        # "k=1;    # label 1\nlab=\"23 mA\";\neval( sprintf (\"set label %d %s\", k, lab))"
        n332 = Strip Path(path=w935) -> (name=w934:string)  [unwired: 1 out]
        n333 = Select(t="2:1", s=w924, f="1:2") -> (s? t:f=w925:string)
        n334 = for {
          tunnel: w937 -> [w953]
          tunnel: w934 -> [w951]
          shift-right: [w949] -> w922
          shift-left: w933 -> [w950]
          tunnel: "Auto Zp" -> [w948]
          tunnel: "Fixed Zp" -> [w947]
          tunnel: w925 -> [w946]
          tunnel: w924 -> [w945]
          tunnel: w923 -> [w944] mode=indexing
          tunnel: [w939] -> w920
          i -> [w952]
          n335 = Unbundle(w944) -> ("Output"=w942:dbl[], "PercentageDifferenceArray"=w940:dbl[])
          n336 = case shown="False" w945 {
            tunnel: [w955 w957] -> w943
            tunnel: w942 -> [w955 w956]
            tunnel: [w954 w956] -> w941
            tunnel: w940 -> [w954 w957]
            frame False {
            }
            frame True {
            }
          }
          n337 = case shown="\"Gauss Lat\"" w953 {
            tunnel: w952 -> [w967 w988 w1003 w1022 w1046 w1050 w1056 w1062 _]
            tunnel: w951 -> [w969 w989 w997 w1027 w1047 w1051 w1057 w1063 _]
            tunnel: w950 -> [w977 w992 w1012 w1037 w1045 w1053 w1059 w1065 w1067]
            tunnel: [w976 w979 w1011 w1036 w1044 w1052 w1058 w1064 w1067] -> w949
            tunnel: w948 -> [_ _ w1002 w1026 _ _ _ _ _]
            tunnel: w947 -> [_ _ w999 w1023 _ _ _ _ _]
            tunnel: w946 -> [w959 w980 w996 w1018 w1043 w1049 w1055 w1061 _]
            tunnel: w943 -> [w960 w981 w995 w1020 _ _ _ _ _]
            tunnel: w941 -> [w961 w982 w994 w1019 _ _ _ _ _]
            tunnel: [w958 w978 w993 w1017 w1042 w1048 w1054 w1060 ""] -> w939
            frame "Gauss Lat" {
              w964 = 0.01  # A value of zero make gnuplot stop working
              w958 = "\nf%d(t) = cmax%d*exp(-((t-offset%d)**2)/(2*sig%d**2))\ncmax%d = %.2f; sig%d = %.2f; offset%d = %.2f           # initial guess for cmax and sig and offset\nfit f%d(t) \"%s.dat\" index %d using %s via cmax%d, sig%d, offset%d #this is a gaussian fit\n"
              n338 = Array Max & Min(array=w961) -> (max value=w971:dbl, max index (indices)=w968:i32)  [unwired: 2 out]
              n339 = Array Max & Min(array=w960) -> (max value=w975:dbl, min value=w974:dbl)  [unwired: 2 out]
              n340 = Index Array(array=w960, index=w968) -> (element=w963:dbl)
              n341 = Subtract(x=w975, y=w974) -> (x-y=w973:dbl)
              n342 = Divide(x=w973, y=6.0) -> (x/y=w970:dbl)
              n343 = Absolute Value(x=w963) -> (abs(x)=w965:dbl)
              n344 = Greater?(x=w965, y=w964) -> (0:w966:bool)
              n345 = Select(t=w963, s=w966, f=w964) -> (s? t:f=w962:dbl)
              n346 = Format Into String(format string=w958, initial string=w977, w967, w967, w967, w967, w967, w971, w967, w970, w967, w962, w967, w969, w967, w959, w967, w967, w967) -> (resulting string=w976:string)  [unwired: 1 in, 1 out]
            }
            frame "Guass glc" {
              w985 = 0.01 ("y")
              w978 = "\nf%d(t) = cmax%d*((t/xmax%d)**(-(1+m%d)*q%d)*exp(((1+m%d)/2)*(1-(t/xmax%d)**(-2*q%d))))\ncmax%d = %.2f; xmax%d = %.2f; m%d = 1;  q%d = 0.73         # initial guess for cmax and xmax q and m\nfit f%d(t) \"%s.dat\" index %d using %s via cmax%d, xmax%d, m%d, q%d  #this is a gaussian fit\n"
              n347 = Array Max & Min(array=w982) -> (max value=w991:dbl, max index (indices)=w990:i32)  [unwired: 2 out]
              n348 = Index Array(array=w981, index=w990) -> (element=w984:dbl)
              n349 = Absolute Value(x=w984) -> (abs(x)=w986:dbl)
              n350 = Greater?(x=w986, y=w985) -> (0:w987:bool)
              n351 = Select(t=w984, s=w987, f=w985) -> (s? t:f=w983:dbl)
              n352 = Format Into String(format string=w978, initial string=w992, w988, w988, w988, w988, w988, w988, w988, w988, w988, w991, w988, w983, w988, w988, w988, w989, w988, w980, w988, w988, w988, w988) -> (resulting string=w979:string)  [unwired: 1 in, 1 out]
            }
            frame "Gauss vert" {
              (unwired) "f1(x) = cmax1*exp(-((x-offset1)**2)/(2*sig1**2))"
              w993 = "\nf%d(t) = cmax%d*(exp(-((t-Zp%d)**2)/(2*sigZ%d**2))+exp(-((t+Zp%d)**2)/(2*sigZ%d**2)))\ncmax%d = %.2f; sigZ%d = %.2f; Zp%d = %.2f           # initial guess for cmax and sig and offset\nfit f%d(t) \"%s.dat\" index %d using %s via cmax%d, sigZ%d%s, Zp%d #this is a gaussian fit\n"
              n353 = Array Max & Min(array=w994) -> (max value=w1006:dbl, max index (indices)=w1004:i32)  [unwired: 2 out]
              n354 = Array Max & Min(array=w995) -> (max value=w1010:dbl, min value=w1009:dbl)  [unwired: 2 out]
              n355 = Index Array(array=w995, index=w1004) -> (element=w1001:dbl)
              n356 = Subtract(x=w1010, y=w1009) -> (x-y=w1008:dbl)
              n357 = Divide(x=w1008, y=6.0) -> (x/y=w1005:dbl)
              n358 = case shown="False" w1002 {
                tunnel: [w1014 w1016] -> w1000
                tunnel: w1001 -> [_ w1016]
                tunnel: w999 -> [w1014 _]
                tunnel: [" #" ""] -> w998
                frame False {
                }
                frame True {
                }
              }
              n359 = Format Into String(format string=w993, initial string=w1012, w1003, w1003, w1003, w1003, w1003, w1003, w1003, w1006, w1003, w1005, w1003, w1000, w1003, w997, w1003, w996, w1003, w1003, w998, w1003) -> (resulting string=w1011:string)  [unwired: 1 in, 1 out]
            }
            frame "Gauss Vert with 2 sig" {
              w1017 = "\nf%d(t) = %s\ncmax%d = %.2f; sigZ_low%d = %.2f; sigZ_up%d = %.2f; Zp%d = %.2f           # initial guess for cmax and sig and offset\nfit f%d(t) \"%s.dat\" index %d using %s via cmax%d, sigZ_low%d, sigZ_up%d%s, Zp%d #this is a gaussian fit\n"
              n360 = Array Max & Min(array=w1019) -> (max value=w1029:dbl, max index (indices)=w1031:i32)  [unwired: 2 out]
              n361 = Array Max & Min(array=w1020) -> (max value=w1035:dbl, min value=w1034:dbl)  [unwired: 2 out]
              n362 = Index Array(array=w1020, index=w1031) -> (element=w1025:dbl)
              n363 = Subtract(x=w1035, y=w1034) -> (x-y=w1033:dbl)
              n364 = Divide(x=w1033, y=6.0) -> (x/y=w1028:dbl)
              n365 = call "Vert_Spread_2_Sig.vi"("Index"=w1022) -> ("resulting string"=w1030:string)
              n366 = case shown="False" w1026 {
                tunnel: [w1039 w1041] -> w1024
                tunnel: w1023 -> [w1039 _]
                tunnel: [" #" ""] -> w1021
                tunnel: w1025 -> [_ w1041]
                frame False {
                }
                frame True {
                }
              }
              n367 = Format Into String(format string=w1017, initial string=w1037, w1022, w1030, w1022, w1029, w1022, w1028, w1022, w1028, w1022, w1024, w1022, w1027, w1022, w1018, w1022, w1022, w1022, w1021, w1022) -> (resulting string=w1036:string)  [unwired: 1 in, 1 out]
            }
            frame "2nd Poly" {
              w1042 = "\nf%d(t) = c%d*t**2 + b%d*t + a%d\n#a%d = 40; b%d = 300; c%d = 1           # initial guess for cmax and sig and offset\nfit f%d(t) \"%s.dat\" index %d using %s via a%d, b%d, c%d #this is a 2nd order poly fit\n"
              n368 = Format Into String(format string=w1042, initial string=w1045, w1046, w1046, w1046, w1046, w1046, w1046, w1046, w1046, w1047, w1046, w1043, w1046, w1046, w1046) -> (resulting string=w1044:string)  [unwired: 1 in, 1 out]
            }
            frame "3rd Poly" {
              w1048 = "\nf%d(t) = d%d*t**3 +c%d*t**2 + b%d*t + a%d\n#a%d = 40; b%d = 300; c%d = 1; d%d = 1         # initial guess for cmax and sig and offset\nfit f%d(t) \"%s.dat\" index %d using %s via a%d, b%d, c%d, d%d #this is a 3rd order poly fit\n"
              n369 = Format Into String(format string=w1048, initial string=w1053, w1050, w1050, w1050, w1050, w1050, w1050, w1050, w1050, w1050, w1050, w1051, w1050, w1049, w1050, w1050, w1050, w1050) -> (resulting string=w1052:string)  [unwired: 1 in, 1 out]
            }
            frame "4th Poly" {
              w1054 = "\nf%d(t) = e%d*t**4 + d%d*t**3 +c%d*t**2 + b%d*t + a%d\n#a%d = 40; b%d = 300; c%d = 1; d%d = 1  e%d = 1       # initial guess for cmax and sig and offset\nfit f%d(t) \"%s.dat\" index %d using %s via a%d, b%d, c%d, d%d, e%d #this is a 3rd order poly fit\n"
              n370 = Format Into String(format string=w1054, initial string=w1059, w1056, w1056, w1056, w1056, w1056, w1056, w1056, w1056, w1056, w1056, w1056, w1056, w1057, w1056, w1055, w1056, w1056, w1056, w1056, w1056) -> (resulting string=w1058:string)  [unwired: 1 in, 1 out]
            }
            frame "Linear" {
              w1060 = "\nf%d(t) = b%d*t + c%d\n#a%d = 40; b%d = 300; c%d = 1           # initial guess for cmax and sig and offset\nfit f%d(t) \"%s.dat\" index %d using %s via b%d, c%d #this is a Linear fit\n"
              n371 = Format Into String(format string=w1060, initial string=w1065, w1062, w1062, w1062, w1062, w1062, w1062, w1062, w1063, w1062, w1061, w1062, w1062) -> (resulting string=w1064:string)  [unwired: 1 in, 1 out]
            }
            frame "Spline", Default {
            }
          }
        }
        n372 = call "ParsingFitFormulae.vi"("String"=w920) -> ("element"=w921:string)
        n373 = local write "Current Fit Formula"(w921) -> ()
        n374 = Concatenate Strings(w922, "save variables 'Coeff.txt'\n") -> (w931:string)
      }
      frame "Edit Legend names" {
        n375 = local read "Profile offset"() -> (w1076:dbl)
        n376 = for {
          tunnel: w1086 -> [w1101] mode=indexing
          tunnel: [w1100] -> w1085 mode=indexing
          tunnel: [w1099] -> w1081
          i -> [w1099]
          n377 = disable-structure shown="Enabled" {
            disable-tunnel: w1101 -> [w1103 w1107]
            disable-tunnel: [w1102 w1107] -> w1094
            frame Disabled {
              n378 = String Length(string=w1103) -> (length=w1106:i32)
              n379 = Subtract(x=w1106, y=2) -> (x-y=w1104:i32)
              n380 = String Subset(string=w1103, length (rest)=w1104) -> (substring=w1102:string)  [unwired: 1 out]
            }
            frame Enabled {
            }
          }
          n381 = Match Pattern(string=w1094, regular expression="=") -> (before substring=w1093:string, match substring=w1092:string, after substring=w1091:string)  [unwired: 2 out]
          n382 = call "Match_Pat_Case_In.vi"("String to match"="legend", "String"=w1093) -> ("offset past match"=w1096:i32)  [unwired: 1 in, 3 out]
          n383 = Greater Than 0?(x=w1096) -> (x > 0?=w1095:bool)
          n384 = case shown="False" w1095 {
            tunnel: [w1108 w1112] -> w1088
            tunnel: w1091 -> [w1109 w1112]
            tunnel: w1093 -> [w1111 _]
            tunnel: w1092 -> [w1110 _]
            frame False {
              n385 = Concatenate Strings(w1111, w1110, w1109) -> (w1108:string)
            }
            frame True {
            }
          }
          n386 = call "Fast_string_Replace.vi"("Replace match with:"=" ", "Input String"=w1088, "matchThis"="_" ("regular expression")) -> ("Output String"=w1087:string)  [unwired: 1 in, 1 out]
          n387 = call "Text_for_latex.vi"("Input String"=w1087) -> ("Output String"=w1100:string)
        }
        n388 = Multiply(x=w1078, y=w1076) -> (x*y=w1080:dbl)
        n389 = Decrement(x=w1078) -> (x-1=w1077:dbl)
        n390 = Multiply(x=w1080, y=w1081) -> (x*y=w1075:dbl)
        n391 = Multiply(x=w1076, y=w1077) -> (x*y=w1074:dbl)
        n392 = Add(x=w1074, y=w1075) -> (x+y=→"Extra range":dbl)
        n393 = Equal To 0?(x="Legend Position") -> (x = 0?=w1071:bool)
        n394 = Select(t="Auto Legend Position", s=w1071, f="Specified Legend Position") -> (s? t:f=w1069:string)
      }
      frame "Auto Legend Position" {
        w1116 = T12 {"Appearance"={"layout"="horizontal", "text-sample order"="", "key order"="", "surroundingBox"="", "MaxRows"=0, "MaxCols"=0, "WidthAdjust"=0.0}, "Alignment"={"Horizontal"="center", "Vertical"="bottom"}, "Location"="", "\"At\" location"={"XcoordSys"="", "YcoordSys"="", "Xvalue"=0.0, "Yvalue"=0.0}}  # LegendProperties
        w1114 = "at"  # Location
        # "Don't know if any of this is really required-  maybe for offset plots.....?"
        n395 = property on="XY Graph" class="XYGraph (strict)"() -> ("X Scale.Range:Maximum"=w1125:dbl, "X Scale.Range:Minimum"=w1124:dbl, "Y Scale.Range:Minimum"=w1128:dbl, "Y Scale.Range:Maximum"=w1126:dbl)  [unwired: 2 in, 2 out]
        n396 = local read "Graph Height"() -> (w1136:string)
        n397 = case shown="True" w1131 {
          tunnel: w1125 -> [w1157 w1161]
          tunnel: w1124 -> [w1156 w1160]
          tunnel: [w1157 w1159] -> w1142
          tunnel: [w1156 w1158] -> w1138
          frame False {
          }
          frame True {
            n398 = Logarithm Base 10(1:w1161) -> (0:w1159:dbl)
            n399 = Logarithm Base 10(1:w1160) -> (0:w1158:dbl)
          }
        }
        n400 = case shown="True" w1134 {
          tunnel: w1126 -> [w1163 w1167]
          tunnel: w1128 -> [w1162 w1166]
          tunnel: [w1163 w1165] -> w1149
          tunnel: [w1162 w1164] -> w1127
          frame False {
          }
          frame True {
            n401 = Logarithm Base 10(1:w1166) -> (0:w1164:dbl)
            n402 = Logarithm Base 10(1:w1167) -> (0:w1165:dbl)
          }
        }
        n403 = local read "Extra range"() -> (w1129:dbl)
        n404 = Fract/Exp String To Number(string=w1136) -> (number=w1135:dbl)  [unwired: 4 out]
        n405 = Subtract(x=w1127, y=w1129) -> (x-y=w1148:dbl)
        n406 = Divide(x=0.35 ("y"), y=w1135) -> (x/y=w1147:dbl)
        n407 = Subtract(x=w1149, y=w1148) -> (x-y=w1145:dbl)
        n408 = Subtract(x=w1142, y=w1138) -> (x-y=w1141:dbl)
        n409 = Multiply(x=w1145, y=w1147) -> (x*y=w1151:dbl)
        n410 = Divide(x=w1145, y=10.0) -> (x/y=w1143:dbl)
        "Delta y" <- w1143
        n411 = Multiply(x=0.9 ("y"), y=w1141) -> (x*y=w1152:dbl)
        n412 = Multiply(x=w1141, y=-0.2 ("x")) -> (x*y=w1139:dbl)
        n413 = Subtract(x=w1148, y=w1151) -> (x-y=w1133:dbl)
        n414 = case shown="True" "Show legend?" {
          tunnel: w1133 -> [w1174 w1180]
          tunnel: [w1174 w1178] -> w1122
          tunnel: w1143 -> [_ w1181]
          frame False {
          }
          frame True {
            n415 = local read "No of Series"() -> (w1177:i32)
            n416 = Add(x=0.65, y=w1177) -> (x+y=w1176:dbl)
            n417 = Multiply(x=w1181, y=w1176) -> (x*y=w1179:dbl)
            n418 = Subtract(x=w1180, y=w1179) -> (x-y=w1178:dbl)
          }
        }
        "Y location" <- w1122
        n419 = Add(x=w1152, y=w1138) -> (x+y=w1132:dbl)
        n420 = Add(x=w1138, y=w1139) -> (x+y=→"X location":dbl)
        n421 = case shown="True" w1131 {
          tunnel: w1132 -> [w1168 w1170]
          tunnel: [w1168 w1169] -> w1120
          frame False {
          }
          frame True {
            n422 = Power Of 10(x=w1170) -> (10^x=w1169:dbl)
          }
        }
        n423 = case shown="True" w1134 {
          tunnel: w1133 -> [w1171 w1173]
          tunnel: [w1171 w1172] -> w1119
          frame False {
          }
          frame True {
            n424 = Power Of 10(x=w1173) -> (10^x=w1172:dbl)
          }
        }
        n425 = local read "Appearance"() -> (w1113:T6)
        n426 = Bundle By Name(cluster=w1116, "\"At\" location.Xvalue"=w1120, "\"At\" location.Yvalue"=w1119, "Location"=w1114, "Appearance"=w1113) -> (w1115:T12)
        n427 = call "setKey.vi"("LegendProperties"=w1115, "Set?"="Show legend?", "String in"=w1121) -> ("String out"=w1118:string)  [unwired: 7 in, 1 out]
      }
      frame "Specified Legend Position" {
        w1186 = T12 {"Appearance"={"layout"="horizontal", "text-sample order"="", "key order"="", "surroundingBox"="", "MaxRows"=0, "MaxCols"=0, "WidthAdjust"=0.0}, "Alignment"={"Horizontal"="center", "Vertical"="bottom"}, "Location"="", "\"At\" location"={"XcoordSys"="", "YcoordSys"="", "Xvalue"=0.0, "Yvalue"=0.0}}  # LegendProperties
        # "Not sure if stuff below is required, to provide \"Y location\"?"
        n428 = property on="XY Graph" class="XYGraph (strict)"() -> ("Y Scale.Range:Minimum"=w1196:dbl, "Y Scale.Range:Maximum"=w1194:dbl)  [unwired: 2 in, 2 out]
        n429 = local read "Graph Height"() -> (w1202:string)
        n430 = case shown="True" w1200 {
          tunnel: w1194 -> [w1215 w1219]
          tunnel: w1196 -> [w1214 w1218]
          tunnel: [w1215 w1217] -> w1208
          tunnel: [w1214 w1216] -> w1195
          frame False {
          }
          frame True {
            n431 = Logarithm Base 10(1:w1219) -> (0:w1217:dbl)
            n432 = Logarithm Base 10(1:w1218) -> (0:w1216:dbl)
          }
        }
        n433 = local read "Extra range"() -> (w1197:dbl)
        n434 = local read "Show legend?"() -> (w1187:bool)
        n435 = Fract/Exp String To Number(string=w1202) -> (number=w1201:dbl)  [unwired: 4 out]
        n436 = Subtract(x=w1195, y=w1197) -> (x-y=w1207:dbl)
        n437 = Divide(x=0.35 ("y"), y=w1201) -> (x/y=w1206:dbl)
        n438 = local read "Legend Position"() -> (w1190:u16)
        n439 = Subtract(x=w1208, y=w1207) -> (x-y=w1205:dbl)
        n440 = property on="Legend Position" class="Ring (strict)"() -> ("Strings []"=w1191:string[])  [unwired: 2 in, 2 out]
        n441 = Multiply(x=w1205, y=w1206) -> (x*y=w1210:dbl)
        n442 = Index Array(array=w1191, index=w1190) -> (element=w1184:string)
        n443 = Divide(x=w1205, y=10.0) -> (x/y=w1203:dbl)
        n444 = Subtract(x=w1207, y=w1210) -> (x-y=w1199:dbl)
        n445 = case shown="True" w1187 {
          tunnel: w1199 -> [w1220 w1226]
          tunnel: [w1220 w1224] -> w1192
          tunnel: w1203 -> [_ w1227]
          frame False {
          }
          frame True {
            n446 = local read "No of Series"() -> (w1223:i32)
            n447 = Add(x=0.65, y=w1223) -> (x+y=w1222:dbl)
            n448 = Multiply(x=w1227, y=w1222) -> (x*y=w1225:dbl)
            n449 = Subtract(x=w1226, y=w1225) -> (x-y=w1224:dbl)
          }
        }
        n450 = Bundle By Name(cluster=w1186, "Location"=w1184, "Appearance"="Appearance", "Alignment"="Alignment") -> (w1185:T12)
        n451 = local write "Y location"(w1192) -> ()
        n452 = call "setKey.vi"("LegendProperties"=w1185, "Set?"=w1187, "String in"=w1189) -> ("String out"=w1188:string)  [unwired: 7 in, 1 out]
      }
      frame "Labels?" {
        n453 = call "setAxisGrids.vi"("Minor Gridlines"="Minor Gridlines", "Major Gridlines"="Major Gridlines", "String in"=w1231) -> ("String out"=w1230:string)  [unwired: 7 in, 1 out]
        n454 = Array Size(array="Added labels") -> (size(s)=w1239:i32)
        n455 = local read "Show Labels?"() -> (w1233:bool)
        n456 = Greater Than 0?(x=w1239) -> (x > 0?=w1235:bool)
        n457 = And(x=w1233, y=w1235) -> (x .and. y?=w1234:bool)
        n458 = Select(t="Add Labels to plot", s=w1234, f="Set plot ranges" ("t")) -> (s? t:f=w1236:string)
      }
      frame "Add Labels to plot" {
        n459 = stacked-sequence {
          seq-local: [w1254 _] -> [_ w1299]
          tunnel: [_ w1300] -> w1251
          tunnel: w1250 -> [_ w1301]
          tunnel: [_ "Set plot ranges" ("t")] -> w1247
          tunnel: w1246 -> [w1257 _]
          tunnel: w1245 -> [_ w1296]
          tunnel: w1244 -> [_ w1294]
          frame #0 {
            n460 = local read "Added labels"() -> (w1259:i32[])
            n461 = Index Array(array=w1257, index (col)=0 ("disabled index (col)")) -> (element=w1258:string[])  [unwired: 1 in]
            n462 = for {
              tunnel: w1259 -> [w1284] mode=indexing
              tunnel: w1258 -> [w1289]
              tunnel: w1257 -> [w1288]
              tunnel: "Summarise" -> [w1287]
              shift-right: [w1275] -> w1254
              shift-left: string[] [] -> [w1276]
              n463 = Add(x=w1287, y=u16 2) -> (x+y=w1285:u16)
              n464 = Index Array(array=w1288, index (col)=w1285) -> (element=w1283:string[])  [unwired: 1 in]
              n465 = Index Array(array=w1289, index=w1284) -> (element=w1280:string)
              n466 = Index Array(array=w1283, index=w1284) -> (element=w1274:string)
              n467 = call "Fast_string_Replace.vi"("Replace match with:"=" ", "Input String"=w1280, "matchThis"=":" ("regular expression")) -> ("Output String"=w1279:string)  [unwired: 1 in, 1 out]
              n468 = call <vilib>:"Trim Whitespace.vi"("string"=w1279) -> ("trimmed string"=w1278:string)  [unwired: 1 in]
              n469 = Match Pattern(string=w1274, regular expression="=") -> (offset past match=w1272:i32)  [unwired: 4 out]
              n470 = Less Than 0?(x=w1272) -> (x < 0?=w1271:bool)
              n471 = Select(t="%s = %s" ("format string"), s=w1271, f="%s %s" ("format string")) -> (s? t:f=w1268:string)
              n472 = Format Into String(format string=w1268, w1278, w1274) -> (resulting string=w1261:string)  [unwired: 2 in, 1 out]
              n473 = Match Pattern(string=w1261, regular expression=";") -> (offset past match=w1266:i32)  [unwired: 4 out]
              n474 = Match Pattern(string=w1261, regular expression=" to ") -> (offset past match=w1265:i32)  [unwired: 4 out]
              n475 = Less Than 0?(x=w1266) -> (x < 0?=w1263:bool)
              n476 = Less Than 0?(x=w1265) -> (x < 0?=w1264:bool)
              n477 = And(x=w1263, y=w1264) -> (x .and. y?=w1262:bool)
              n478 = case shown="False" w1262 {
                tunnel: w1276 -> [w1290 w1293]
                tunnel: [w1290 w1291] -> w1275
                tunnel: w1261 -> [_ w1292]
                frame False {
                }
                frame True {
                  n479 = Build Array (concatenate)(w1293, w1292) -> (w1291:string[])
                }
              }
            }
          }
          frame #1 {
            n480 = local read "Show legend?"() -> (w1295:bool)
            n481 = local read "X location"() -> (w1298:dbl)
            n482 = local read "Delta y"() -> (w1297:dbl)
            n483 = for {
              shift-right: [w1322] -> w1300
              shift-left: w1301 -> [w1323]
              tunnel: w1299 -> [w1319] mode=indexing
              tunnel: w1298 -> [w1305]
              tunnel: w1297 -> [w1324]
              tunnel: w1296 -> [w1318]
              tunnel: w1295 -> [w1307]
              tunnel: w1294 -> [w1303]
              i -> [w1325]
              n484 = call "Text_for_latex.vi"("Input String"=w1319) -> ("Output String"=w1313:string)
              n485 = case shown="False" w1303 {
                tunnel: w1305 -> [w1328 w1330]
                tunnel: [w1328 w1329] -> w1304
                frame False {
                }
                frame True {
                  n486 = Power Of 10(x=w1330) -> (10^x=w1329:dbl)
                }
              }
              n487 = String Length(string=w1313) -> (length=w1316:i32)
              n488 = Less?(x=w1316, y=20) -> (x < y?=w1308:bool)
              n489 = Compound Arithmetic op=AND(w1308, invert w1307) -> (w1306:bool)
              n490 = Increment(x=w1325) -> (x+1=w1326:i32)
              n491 = case shown="True" w1306 {
                tunnel: [w1331 w1333] -> w1314
                tunnel: w1313 -> [w1331 w1334]
                tunnel: "~~~~~~~~~~~" -> [_ w1332]
                frame False {
                }
                frame True {
                  n492 = Concatenate Strings(w1332, w1334) -> (w1333:string)
                }
              }
              n493 = Multiply(x=w1325, y=w1324) -> (x*y=w1320:dbl)
              n494 = local read "Y location"() -> (w1321:dbl)
              n495 = call "Number_2_string.vi"("number"=w1304) -> ("String"=w1311:string)  [unwired: 1 in]
              n496 = Subtract(x=w1321, y=w1320) -> (x-y=w1317:dbl)
              n497 = case shown="False" w1318 {
                tunnel: w1317 -> [w1335 w1337]
                tunnel: [w1335 w1336] -> w1310
                frame False {
                }
                frame True {
                  n498 = Power Of 10(x=w1337) -> (10^x=w1336:dbl)
                }
              }
              n499 = call "Number_2_string.vi"("number"=w1310) -> ("String"=w1309:string)  [unwired: 1 in]
              n500 = Format Into String(format string="set label %d '%s' at %s, %s\n", initial string=w1323, w1326, w1314, w1311, w1309) -> (resulting string=w1322:string)  [unwired: 1 in, 1 out]
            }
          }
        }
      }
      frame "Set plot ranges" {
        w1338 = ""
        (unwired) "set border"
        (unwired) "set nologscale  y"
        (unwired) "set logscale  y"
        w1340 = "#"
        w1342 = ""
        n501 = local read "Profile offset"() -> (w1365:dbl)
        n502 = property on="XY Graph" class="XYGraph (strict)"() -> ("X Scale.Range:Maximum"=w1375:dbl, "X Scale.Range:Minimum"=w1374:dbl, "Y Scale.Range:Maximum"=w1358:dbl, "Y Scale.Range:Minimum"=w1359:dbl)  [unwired: 2 in, 2 out]
        n503 = local read "Extra range"() -> (w1369:dbl)
        n504 = Decrement(x=w1364) -> (x-1=w1366:dbl)
        n505 = Multiply(x=w1365, y=w1366) -> (x*y=w1363:dbl)
        n506 = Add(x=w1363, y=w1358) -> (x+y=w1362:dbl)
        n507 = Subtract(x=w1359, y=w1369) -> (x-y=w1370:dbl)
        n508 = call "Number_2_string.vi"("number"=w1362) -> ("String"=w1347:string)  [unwired: 1 in]
        n509 = call "Gnuplot_offset_ytics.vi"("Separation"=w1364, "Mode"="Mode", "precision"="precision", "Legend"=w1367, "Max Plot Value"=w1358, "Profile offset"=w1365) -> ("concatenated string"=w1354:string)
        n510 = call "Number_2_string.vi"("number"=w1375) -> ("String"=w1349:string)  [unwired: 1 in]
        n511 = call "Number_2_string.vi"("number"=w1374) -> ("String"=w1350:string)  [unwired: 1 in]
        n512 = call "Number_2_string.vi"("number"=w1370) -> ("String"=w1348:string)  [unwired: 1 in]
        n513 = case shown="True" w1351 {
          tunnel: [w1387 w1389] -> w1345
          tunnel: w1350 -> [w1387 _]
          tunnel: [w1386 w1388] -> w1344
          tunnel: w1349 -> [w1386 _]
          tunnel: w1348 -> [_ w1389]
          tunnel: w1347 -> [_ w1388]
          frame False {
          }
          frame True {
          }
        }
        n514 = local read "Time format?"() -> (w1339:bool)
        n515 = Select(t="\nset logscale  x\n", s=w1356, f=w1342) -> (s? t:f=w1353:string)
        n516 = Select(t="\nset logscale  y\n", s=w1361, f=w1342) -> (s? t:f=w1355:string)
        n517 = case shown="\"Linear\", Default" w1346 {
          tunnel: w1345 -> [_ w1384]
          tunnel: w1344 -> [_ w1383]
          tunnel: ["" w1382] -> w1343
          frame "Spline" {
          }
          frame "Linear", Default {
            n518 = Format Into String(format string="set trange [%s : %s]", w1384, w1383) -> (resulting string=w1382:string)  [unwired: 2 in, 1 out]
          }
        }
        n519 = Select(t=w1338, s=w1339, f=w1340) -> (s? t:f=w1341:string)
        n520 = Format Into String(format string="%s set xrange [%s : %s] \n%s set autoscale x \n%s set yrange [%s : %s]\n%s set autoscale y\n", initial string=w1377, w1338, w1350, w1349, w1341, w1338, w1348, w1347, w1340) -> (resulting string=w1372:string)  [unwired: 1 in, 1 out]
        n521 = Concatenate Strings(w1372, w1343, w1353, w1355, w1354) -> (w1373:string)
      }
      frame "Plot Command" {
        n522 = case shown="True" w1399 {
          tunnel: ["yerrorbars" "xerrorbars"] -> w1398
          tunnel: ["" ", t"] -> w1397
          tunnel: ["t, " ""] -> w1396
          frame False {
          }
          frame True {
          }
        }
        n523 = Strip Path(path=w1411) -> (name=w1393:string)  [unwired: 1 out]
        n524 = Format Into String(format string="\nfile=\"%s.dat\"\n\nplot ", w1393) -> (resulting string=w1394:string)  [unwired: 2 in, 1 out]
        n525 = global read "Results_plotter_Global.vi" "Series Index"() -> (w1400:i32[])
        n526 = for {
          shift-right: [w1457] -> w1392
          shift-left: w1394 -> [w1458]
          tunnel: w1405 -> [w1456]
          tunnel: w1410 -> [w1451] mode=indexing
          tunnel: "Plot style" -> [w1452]
          tunnel: w1403 -> [w1439]
          tunnel: w1402 -> [w1450] mode=indexing
          tunnel: "plot error bars?" -> [w1446]
          tunnel: w1398 -> [w1430]
          tunnel: w1400 -> [w1423] mode=indexing
          tunnel: w1397 -> [w1426]
          tunnel: w1396 -> [w1425]
          tunnel: "Fit Line Width" -> [w1419]
          i -> [w1427]
          n527 = Index Array(array=w1452, index=w1423) -> (element=w1434:u16)
          n528 = Quotient & Remainder(x=w1423, y=8) -> (x-y*floor(x/y)=w1438:i32)  [unwired: 1 out]
          n529 = call "Fast_string_Replace.vi"("Replace match with:"="", "Input String"=w1451, "matchThis"="[$]" ("regular expression")) -> ("Output String"=w1441:string)  [unwired: 1 in, 1 out]
          n530 = case shown="2" w1434 {
            tunnel: ["points" ("format string") "lines" ("format string") "linespoints" ("format string")] -> w1431
            frame 0, Default {
            }
            frame 1 {
            }
            frame 2 {
            }
          }
          n531 = case shown="\"Spline\"" w1456 {
            tunnel: w1427 -> [_ w1469 w1476 w1483 w1490 w1498 w1505 w1512 w1519 w1526]
            tunnel: ["" w1470 w1477 w1484 w1492 w1499 w1506 w1513 w1520 w1527] -> w1455
            tunnel: w1423 -> [_ w1468 w1475 w1481 w1489 w1497 w1504 w1511 w1518 w1525]
            tunnel: "Fit Line Type" -> [_ w1467 w1474 w1482 w1488 w1496 w1503 w1510 w1517 w1524]
            tunnel: w1426 -> [_ _ w1472 w1480 w1486 w1494 w1501 w1508 w1515 w1522]
            tunnel: w1425 -> [_ _ w1473 w1479 w1487 w1495 w1502 w1509 w1516 w1523]
            tunnel: w1419 -> [_ w1466 _ _ _ _ _ _ _ _]
            frame "None", Default {
            }
            frame "Spline" {
              n532 = Format Into String(format string="file index %d using 1:2 axes x1y1 title'' linecolor %d lw %d linetype %d  smooth csplines, ", w1469, w1468, w1466, w1467) -> (resulting string=w1470:string)  [unwired: 2 in, 1 out]
            }
            frame "Gauss Lat" {
              n533 = Format Into String(format string="%s cmax%d*exp(-((t-offset%d)**2)/(2*sig%d**2))%s  linecolor %d linetype %d title '', ", w1473, w1476, w1476, w1476, w1472, w1475, w1474) -> (resulting string=w1477:string)  [unwired: 2 in, 1 out]
            }
            frame "Gauss vert" {
              n534 = Format Into String(format string="%s cmax%d*(exp(-((t-Zp%d)**2)/(2*sigZ%d**2))+exp(-((t+Zp%d)**2)/(2*sigZ%d**2)))%s linecolor %d linetype %d title '', ", w1479, w1483, w1483, w1483, w1483, w1483, w1480, w1481, w1482) -> (resulting string=w1484:string)  [unwired: 2 in, 1 out]
            }
            frame "Gauss Vert with 2 sig" {
              n535 = call "Vert_Spread_2_Sig.vi"("Index"=w1490) -> ("resulting string"=w1491:string)
              n536 = Format Into String(format string="%s %s%s  linecolor %d linetype %d title '', ", w1487, w1491, w1486, w1489, w1488) -> (resulting string=w1492:string)  [unwired: 2 in, 1 out]
            }
            frame "Guass glc" {
              n537 = Format Into String(format string="%s cmax%d*((t/xmax%d)**(-(1+m%d)*q%d)*exp(((1+m%d)/2)*(1-(t/xmax%d)**(-2*q%d))))%s  linecolor %d linetype %d title '', ", w1495, w1498, w1498, w1498, w1498, w1498, w1498, w1498, w1494, w1497, w1496) -> (resulting string=w1499:string)  [unwired: 2 in, 1 out]
            }
            frame "2nd Poly" {
              n538 = Format Into String(format string="%s c%d*t**2 + b%d*t + a%d%s  linecolor %d linetype %d title 'fit%d', ", w1502, w1505, w1505, w1505, w1501, w1504, w1503, w1505) -> (resulting string=w1506:string)  [unwired: 2 in, 1 out]
            }
            frame "3rd Poly" {
              n539 = Format Into String(format string="%s d%d*t**3  + c%d*t**2 + b%d*t + a%d %s linecolor %d linetype %d title 'fit%d', ", w1509, w1512, w1512, w1512, w1512, w1508, w1511, w1510, w1512) -> (resulting string=w1513:string)  [unwired: 2 in, 1 out]
            }
            frame "4th Poly" {
              n540 = Format Into String(format string="%s e%d*t**4 + d%d*t**3  + c%d*t**2 + b%d*t + a%d%s  linecolor %d linetype %d title 'fit%d', ", w1516, w1519, w1519, w1519, w1519, w1519, w1515, w1518, w1517, w1519) -> (resulting string=w1520:string)  [unwired: 2 in, 1 out]
            }
            frame "Linear" {
              n541 = Format Into String(format string="%s b%d*t + c%d%s  linecolor %d linetype %d title 'fit%d', ", w1523, w1526, w1526, w1522, w1525, w1524, w1526) -> (resulting string=w1527:string)  [unwired: 2 in, 1 out]
            }
          }
          n542 = Index Array(array=w1439, index=w1438) -> (element=w1421:i32)
          n543 = case shown="True" "Black and white?" {
            tunnel: w1423 -> [w1460 _]
            tunnel: [w1460 0] -> w1422
            frame False {
            }
            frame True {
            }
          }
          n544 = Unbundle(w1450) -> ("Upper"=w1449:string[])  [unwired: 2 out]
          n545 = Array Size(array=w1449) -> (size(s)=w1448:i32)
          n546 = Greater Than 0?(x=w1448) -> (x > 0?=w1447:bool)
          n547 = And(x=w1447, y=w1446) -> (x .and. y?=w1432:bool)
          n548 = Select(t=w1430, s=w1432, f=w1431) -> (s? t:f=w1429:string)
          n549 = Select(t=":3", s=w1432, f="") -> (s? t:f=w1442:string)
          n550 = Format Into String(format string="file index %d using 1:2%s axes x1y1 title '$%s$' with ", initial string=w1458, w1427, w1442, w1441) -> (resulting string=w1445:string)  [unwired: 1 in, 1 out]
          n551 = Format Into String(format string=" linecolor %d pointtype %d pointsize %.2f linetype %d, ", initial string=w1429, w1422, w1421, "Point Size", w1421) -> (resulting string=w1433:string)  [unwired: 1 in, 1 out]
          n552 = Concatenate Strings(w1445, w1433, w1455, "\\" ("string"), "\n") -> (w1457:string)
        }
        n553 = call "removeLastContinuation.vi"("String in"=w1392) -> ("String out"=w1391:string)  [unwired: 10 in]
        n554 = Concatenate Strings(w1409, w1391) -> (w1408:string)
      }
      frame "Write gnuplot file" {
        w1537 = FALSE  # append to file? (new file:F)
        w1538 = FALSE  # advisory dialog? (display:T)
        n555 = Strip Path(path=w1534) -> (stripped path=w1530:path)  [unwired: 1 out]
        n556 = Build Path(base path=w1530, name or relative path="gnuplot_script.txt") -> (appended path=w1539:path)
        n557 = call "gnuplot_legend.vi"("Plot style"=w1531, "Legend"=w1535) -> ()  [unwired: 1 out]
        n558 = call "Write_Characters_To_File.vi"("file path (dialog if empty)"=w1539, "advisory dialog? (display:T)"=w1538, "character string"=w1529, "append to file? (new file:F)"=w1537) -> ()  [unwired: 1 in, 4 out]
      }
      frame "Execute shell script" {
        n559 = call "Run_Gnuplot_Script.vi"("logfileName"=w1541, "targetFile"=w1542) -> ()  [unwired: 1 in]
      }
      frame "Has pdf been generated?" {
        n560 = Strip Path(path=w1555) -> (stripped path=w1557:path, name=w1559:string)
        n561 = Concatenate Strings(w1559, ".pdf" ("string")) -> (w1558:string)
        n562 = Build Path(base path=w1557, name or relative path=w1558) -> (appended path=w1554:path)
        n563 = call "Does_file_exist_(simple).vi"("Pathname"=w1554) -> ("exists?"=w1553:bool)
        n564 = case shown="False" w1553 {
          tunnel: ["Open Standard output file" ("f") "Input Fit Coefficients into results file?"] -> w1548
          frame False {
          }
          frame True {
          }
        }
        n565 = Select(t="Show Re-Run Gnuplot?", s="Show Re-Run Gnuplot?", f=w1548) -> (s? t:f=w1549:string)
      }
      frame "Show Re-Run Gnuplot?" {
        n566 = Strip Path(path=w1566) -> (stripped path=w1565:path)  [unwired: 1 out]
        n567 = call "Re_run_Gnuplot.vi"("Plot folder (dialog if empty)"=w1565) -> ()  [unwired: 1 in, 3 out]
      }
      frame "Input Fit Coefficients into results file?" {
        n568 = Greater?(x=w1576, y=T4."Spline" ("Fit type")) -> (0:w1575:bool)
        n569 = And(x="Put Coeff\nin Results file", y=w1575) -> (x .and. y?=w1573:bool)
      }
      frame "Read Fit Coefficients" {
        n570 = call "Fast_string_Replace.vi"("Replace match with:"="", "Input String"=w1587, "matchThis"=":" ("regular expression")) -> ("Output String"=w1586:string)  [unwired: 1 in, 1 out]
        n571 = Strip Path(path=w1599) -> (stripped path=w1597:path)  [unwired: 1 out]
        n572 = Build Path(base path=w1597, name or relative path="Coeff.txt") -> (appended path=w1596:path)
        n573 = call "Read_File_Simple.vi"("Filename"=w1596) -> ("string"=w1594:string)  [unwired: 2 in, 7 out]
        n574 = global read "Results_plotter_Global.vi" "Plot Metadata"() -> (w1583:T14[])
        n575 = case shown="True" w1585 {
          tunnel: [w1604 w1605] -> w1584
          tunnel: w1583 -> [w1604 w1606]
          frame False {
          }
          frame True {
            n576 = Reverse 1D Array(array=w1606) -> (reversed array=w1605:T14[])
          }
        }
        n577 = for {
          tunnel: w1595 -> [w1628]
          tunnel: w1594 -> [w1627]
          tunnel: [w1617] -> w1593
          tunnel: w1592 -> [w1625] mode=indexing
          shift-right: [w1622] -> w1590
          shift-left: string[][] [] -> [w1623]
          tunnel: w1586 -> [w1609]
          tunnel: w1584 -> [w1608] mode=indexing
          tunnel: [w1607] -> w1582 mode=concatenating
          i -> [w1619]
          n578 = case shown="\"Gauss Lat\"" w1628 {
            tunnel: w1619 -> [_ w1654 w1667 w1678 w1682 w1699 w1713]
            tunnel: [string[] [] w1650 w1663 w1675 w1690 w1705 w1717] -> w1616
            tunnel: [string[] [] w1646 w1659 w1672 w1687 w1702 w1716] -> w1626
            frame "None", Default {
            }
            frame "Gauss Lat" {
              n579 = Format Into String(format string="sig%d", w1654) -> (resulting string=w1652:string)  [unwired: 2 in, 1 out]
              n580 = Format Into String(format string="offset%d", w1654) -> (resulting string=w1651:string)  [unwired: 2 in, 1 out]
              n581 = Format Into String(format string="cmax%d", w1654) -> (resulting string=w1653:string)  [unwired: 2 in, 1 out]
              n582 = Build Array(":Max:Lat", ":Sig Y:", ":Yo:", ":FitFormula:Lat") -> (w1646:string[])
              n583 = Build Array(w1653, w1652, w1651) -> (w1650:string[])
            }
            frame "2nd Poly" {
              n584 = Format Into String(format string="b%d", w1667) -> (resulting string=w1665:string)  [unwired: 2 in, 1 out]
              n585 = Format Into String(format string="c%d", w1667) -> (resulting string=w1664:string)  [unwired: 2 in, 1 out]
              n586 = Format Into String(format string="a%d", w1667) -> (resulting string=w1666:string)  [unwired: 2 in, 1 out]
              n587 = Build Array(":Coeff:A", ":Coeff:B", ":Coeff:C", ":FitFormula:Poly2") -> (w1659:string[])
              n588 = Build Array(w1666, w1665, w1664) -> (w1663:string[])
            }
            frame "Linear" {
              n589 = Format Into String(format string="c%d", w1678) -> (resulting string=w1677:string)  [unwired: 2 in, 1 out]
              n590 = Format Into String(format string="b%d", w1678) -> (resulting string=w1676:string)  [unwired: 2 in, 1 out]
              n591 = Build Array(":Offset:A", ":Grad:B", ":FitFormula:Lin") -> (w1672:string[])
              n592 = Build Array(w1677, w1676) -> (w1675:string[])
            }
            frame "Gauss Vert with 2 sig" {
              n593 = Format Into String(format string="Zp%d", w1682) -> (resulting string=w1691:string)  [unwired: 2 in, 1 out]
              n594 = Format Into String(format string="cmax%d", w1682) -> (resulting string=w1693:string)  [unwired: 2 in, 1 out]
              n595 = Format Into String(format string="sigZ_low%d", w1682) -> (resulting string=w1683:string)  [unwired: 2 in, 1 out]
              n596 = Format Into String(format string="sigZ_up%d", w1682) -> (resulting string=w1692:string)  [unwired: 2 in, 1 out]
              n597 = Build Array(":Max:Vert", ":Sig Z:Upper", ":Sig Z:Lower", ":Zp:", ":FitFormula:Vert2sig") -> (w1687:string[])
              n598 = Build Array(w1693, w1692, w1683, w1691) -> (w1690:string[])
            }
            frame "Gauss vert" {
              n599 = Format Into String(format string="Zp%d", w1699) -> (resulting string=w1706:string)  [unwired: 2 in, 1 out]
              n600 = Format Into String(format string="cmax%d", w1699) -> (resulting string=w1707:string)  [unwired: 2 in, 1 out]
              n601 = Format Into String(format string="sigZ%d", w1699) -> (resulting string=w1698:string)  [unwired: 2 in, 1 out]
              n602 = Build Array(":Max:Vert", ":Sig Z:Upper", ":Sig Z:Lower", ":Zp:", ":FitFormula:Vert") -> (w1702:string[])
              n603 = Build Array(w1707, w1698, w1698, w1706) -> (w1705:string[])
            }
            frame "Guass glc" {
              n604 = Format Into String(format string="xmax%d", w1713) -> (resulting string=w1722:string)  [unwired: 2 in, 1 out]
              n605 = Format Into String(format string="m%d", w1713) -> (resulting string=w1721:string)  [unwired: 2 in, 1 out]
              n606 = Format Into String(format string="q%d", w1713) -> (resulting string=w1712:string)  [unwired: 2 in, 1 out]
              n607 = Format Into String(format string="cmax%d", w1713) -> (resulting string=w1723:string)  [unwired: 2 in, 1 out]
              n608 = Build Array(":MaxC:glc", ":MaxX:glc", ":m:glc", ":q:glc", ":FitFormula:glc") -> (w1716:string[])
              n609 = Build Array(w1723, w1722, w1721, w1712) -> (w1717:string[])
            }
          }
          n610 = global read "Results_plotter_Global.vi" "Full Ch Names"() -> (w1611:string[])
          n611 = global read "Results_plotter_Global.vi" "Absisca"() -> (w1612:i32)
          n612 = Index Array(array=w1611, index=w1612) -> (element=w1610:string)
          n613 = for {
            tunnel: w1609 -> [w1636]
            tunnel: w1626 -> [w1635] mode=indexing
            tunnel: [w1634] -> w1617 mode=indexing
            n614 = Concatenate Strings(w1636, w1635) -> (w1634:string)
          }
          n615 = Unbundle(w1625) -> ("Output"=w1620:dbl[])  [unwired: 1 out]
          n616 = Array Size(array=w1620) -> (size(s)=w1621:i32)
          n617 = for {
            tunnel: w1616 -> [w1642] mode=indexing
            tunnel: w1627 -> [w1639]
            tunnel: [w1637] -> w1615 mode=indexing
            n618 = Concatenate Strings(w1642, " = " ("string")) -> (w1640:string)
            n619 = Match Pattern(string=w1639, regular expression=w1640) -> (after substring=w1638:string)  [unwired: 4 out]
            n620 = call "Split_at_return.vi"("String"=w1638) -> ("before substring"=w1637:string)  [unwired: 1 in, 3 out]
          }
          n621 = call "ReformatFitFormula.vi"("Current Fit Formula"="Current Fit Formula", "Curve Fit Index"=w1619, "Variables"=w1616, "Channel Names"=w1617, "X Axis Full Ch Name"=w1610) -> ("Reformatted Current Fit Formula"=w1614:string)
          n622 = disable-structure shown="Enabled" {
            disable-tunnel: w1615 -> [w1631 w1632]
            disable-tunnel: w1614 -> [w1630 _]
            disable-tunnel: [w1629 w1632] -> w1613
            frame Enabled {
              n623 = Build Array (concatenate)(w1631, w1630) -> (w1629:string[])
            }
            frame Disabled {
            }
          }
          n624 = for {
            N: w1621 -> [_]
            tunnel: w1613 -> [w1633]
            tunnel: [w1633] -> w1624 mode=indexing
          }
          n625 = Unbundle By Name(w1608) -> ("Row Number"=w1607:i32[])
          n626 = Build Array (concatenate)(w1623, w1624) -> (w1622:string[][])
        }
        n627 = global write "Results_plotter_Global.vi" "New Values Row index"(w1582) -> ()
        n628 = global write "Results_plotter_Global.vi" "New Values In"(w1590) -> ()
        n629 = global write "Results_plotter_Global.vi" "New Chs In"(w1593) -> ()
      }
      frame "Open Standard output file" {
        n630 = Strip Path(path=w1731) -> (stripped path=w1728:path)  [unwired: 1 out]
        n631 = Format Into String(format string="open \"%s\"", w1729) -> (resulting string=w1727:string)  [unwired: 2 in, 1 out]
        n632 = call <vilib>:"System Exec.vi"("working directory"=w1728, "command line"=w1727) -> ()  [unwired: 4 in, 6 out]
      }
    }
  }
  "Tex Info String" <- w18
  "Saved Automatically?" <- FALSE
